vi "QuizPrimeroFinal.vi"() -> ()   [LabVIEW 2020]
panel:
  in  "?":bool
  out "El contador se encuentra":dbl
  out "LED3":bool
  out "LED2":bool
  out "LED1":bool
  out "SW/CO":bool
  out "Led Tres":bool
  out "Led Dos":bool
  out "Led Uno":bool
  in  "Pulsador Tres":bool
  in  "Pulsador Dos":bool
  in  "Pulsador Uno":bool
  out "Visualizador del tiempo del contador en ms":i32
  out "Contador del sistema":dbl
  out "Respuesta de la trama":string
  in  "Ingrese la trama completa":string
  in  "Botón ENTER":bool
  out "Respuesta de comandos":string
  out "Opción":i8
  in  "Ingrese comando":string
  # "Comandos AT"
  # "Indicadores"
  # "Botón STOP"
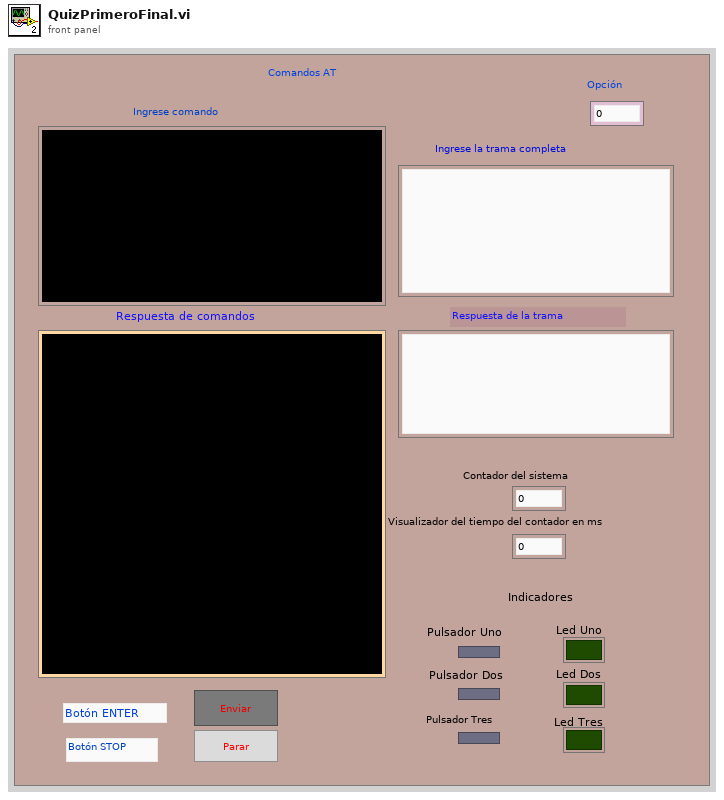
[diagram p1: front panel]
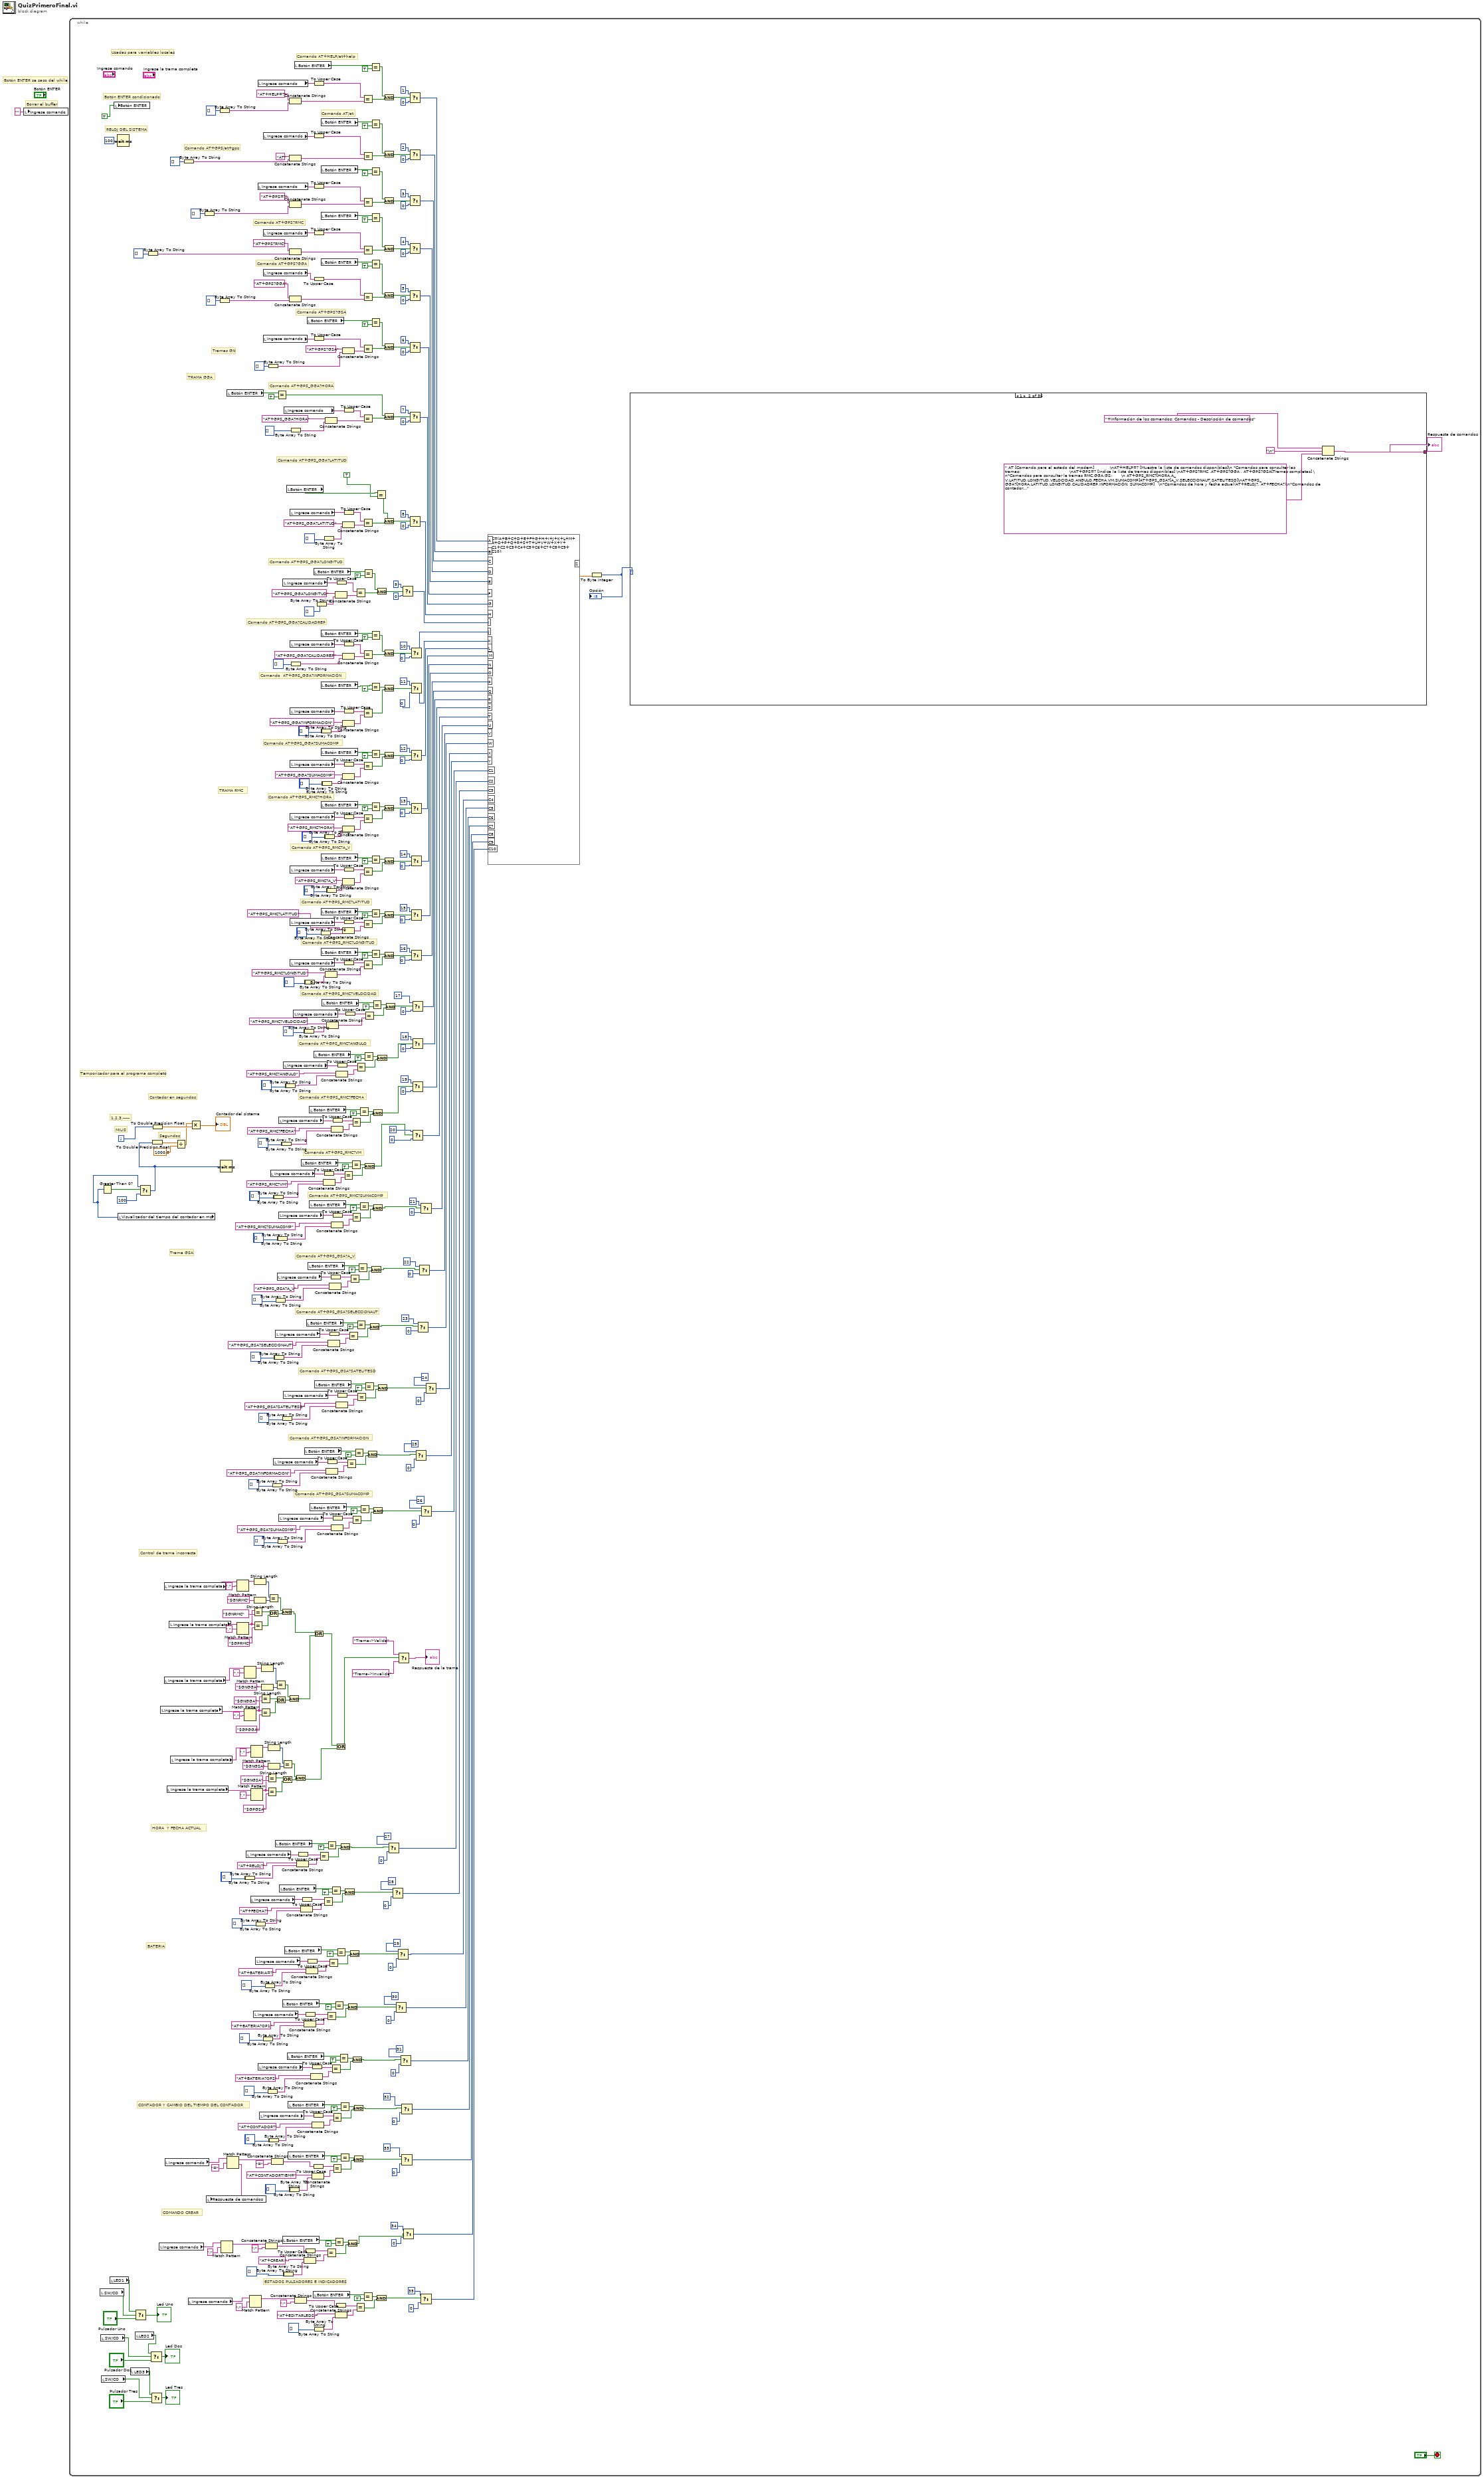
[diagram p0: block diagram]
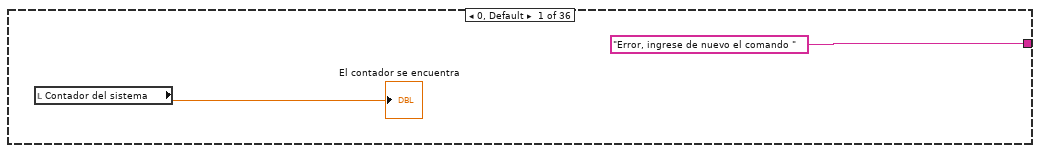
[diagram p2: hidden frame]
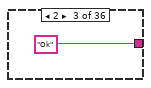
[diagram p3: hidden frame]
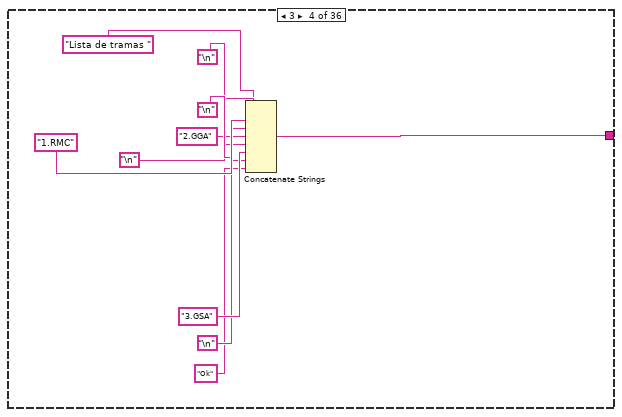
[diagram p4: hidden frame]
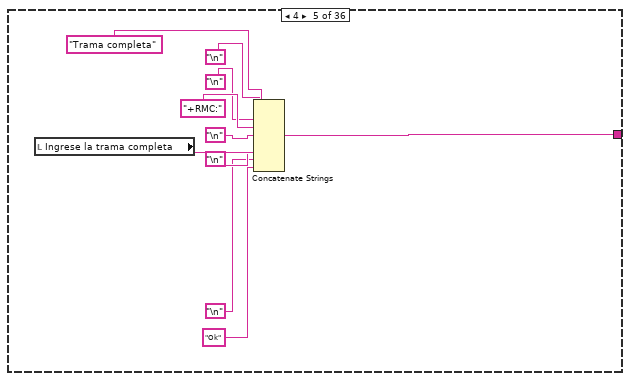
[diagram p5: hidden frame]
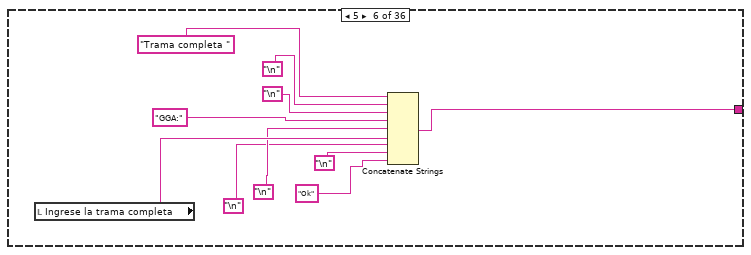
[diagram p6: hidden frame]
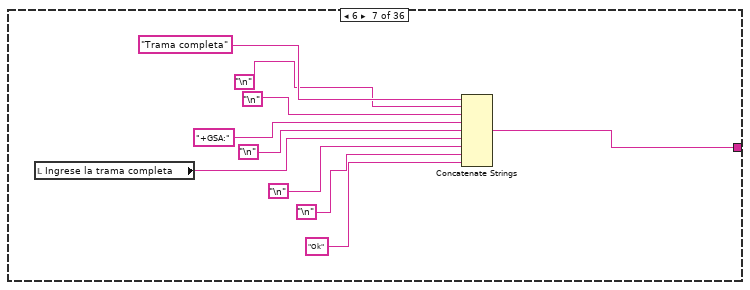
[diagram p7: hidden frame]
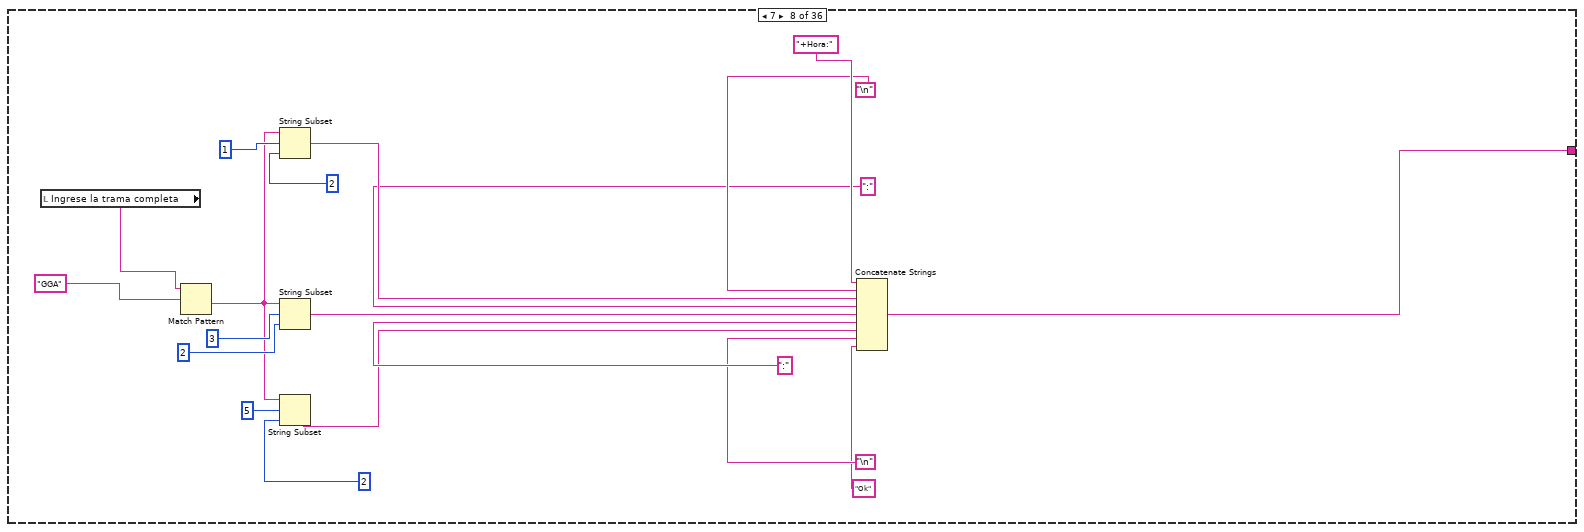
[diagram p8: hidden frame]
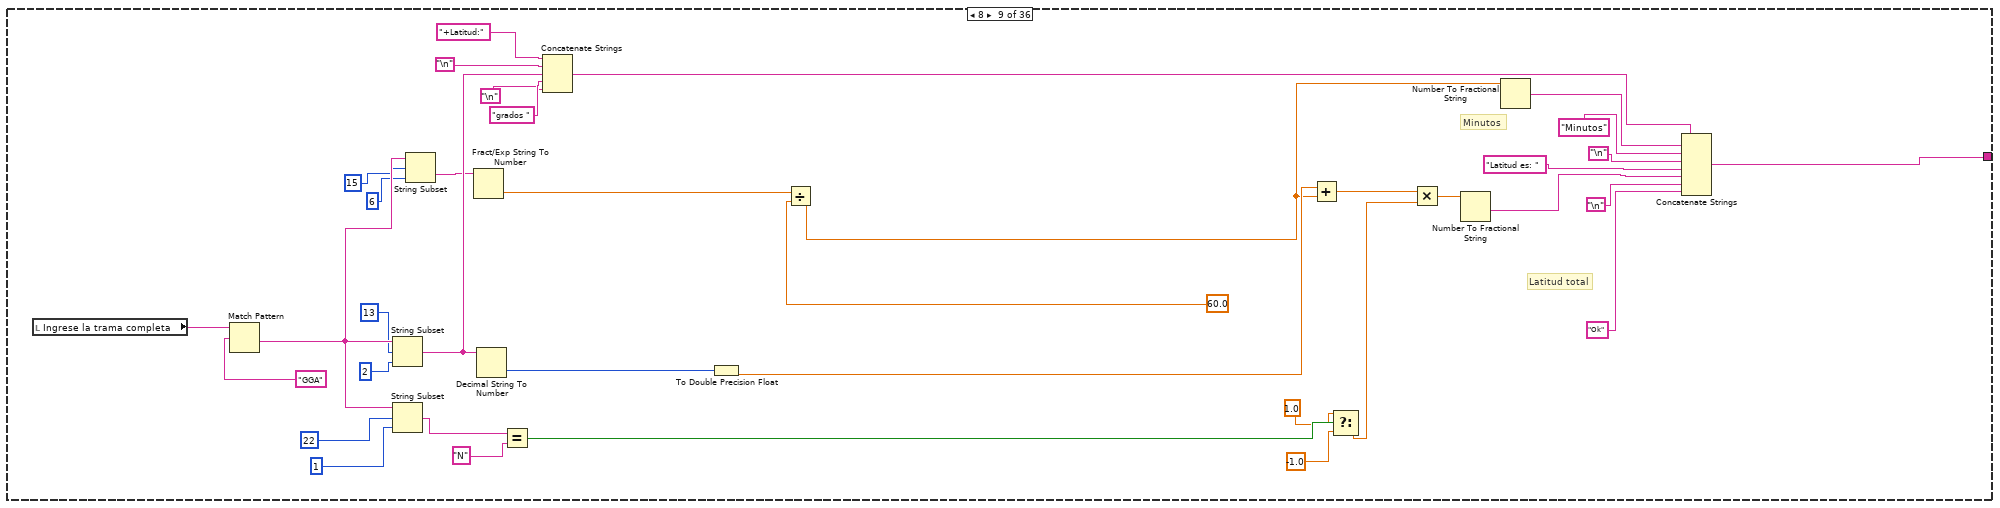
[diagram p9: hidden frame]
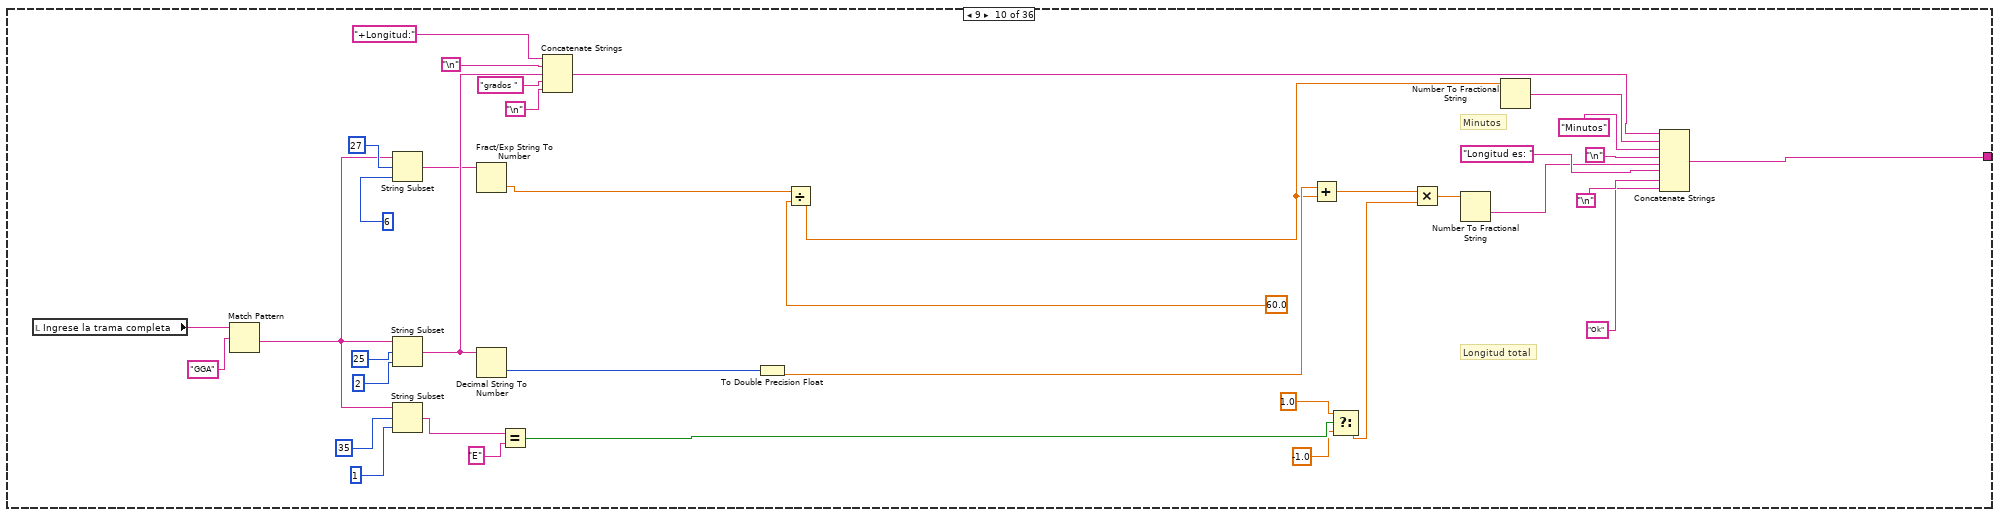
[diagram p10: hidden frame]
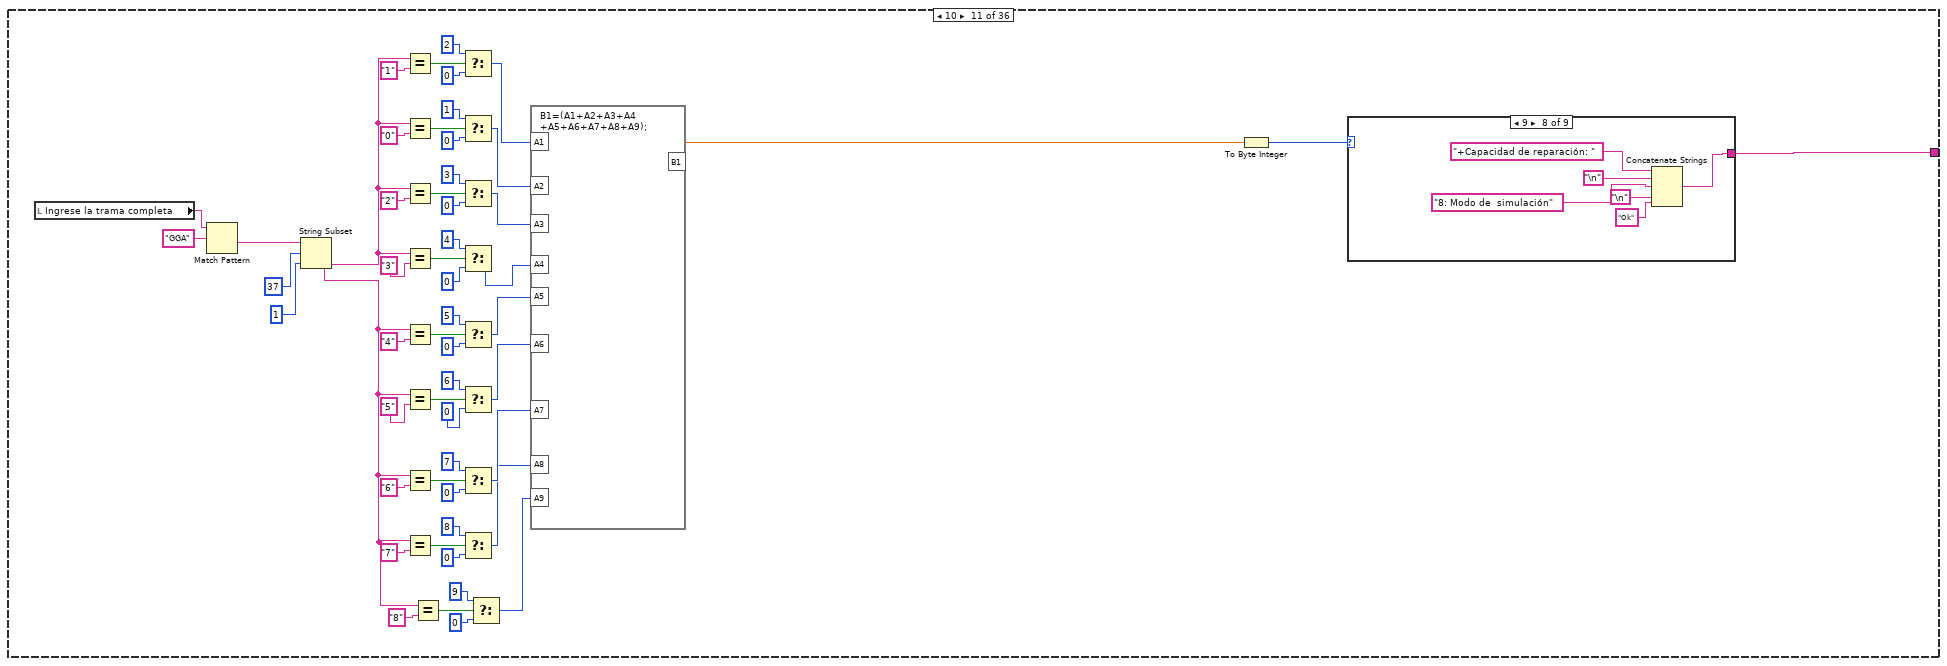
[diagram p11: hidden frame]
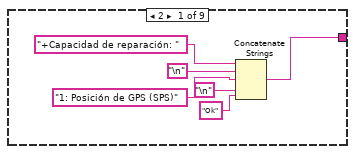
[diagram p12: hidden frame]
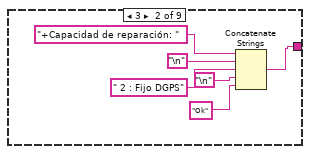
[diagram p13: hidden frame]
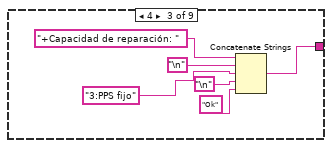
[diagram p14: hidden frame]
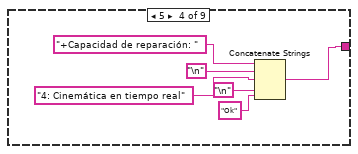
[diagram p15: hidden frame]
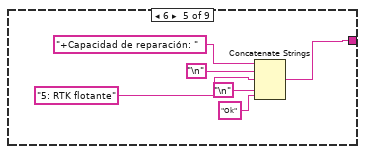
[diagram p16: hidden frame]
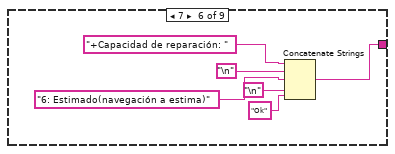
[diagram p17: hidden frame]
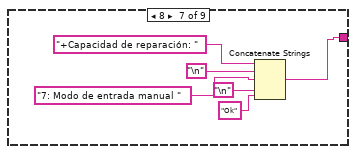
[diagram p18: hidden frame]
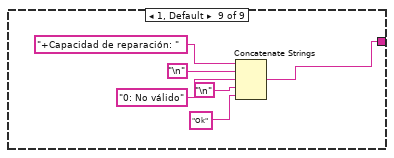
[diagram p19: hidden frame]
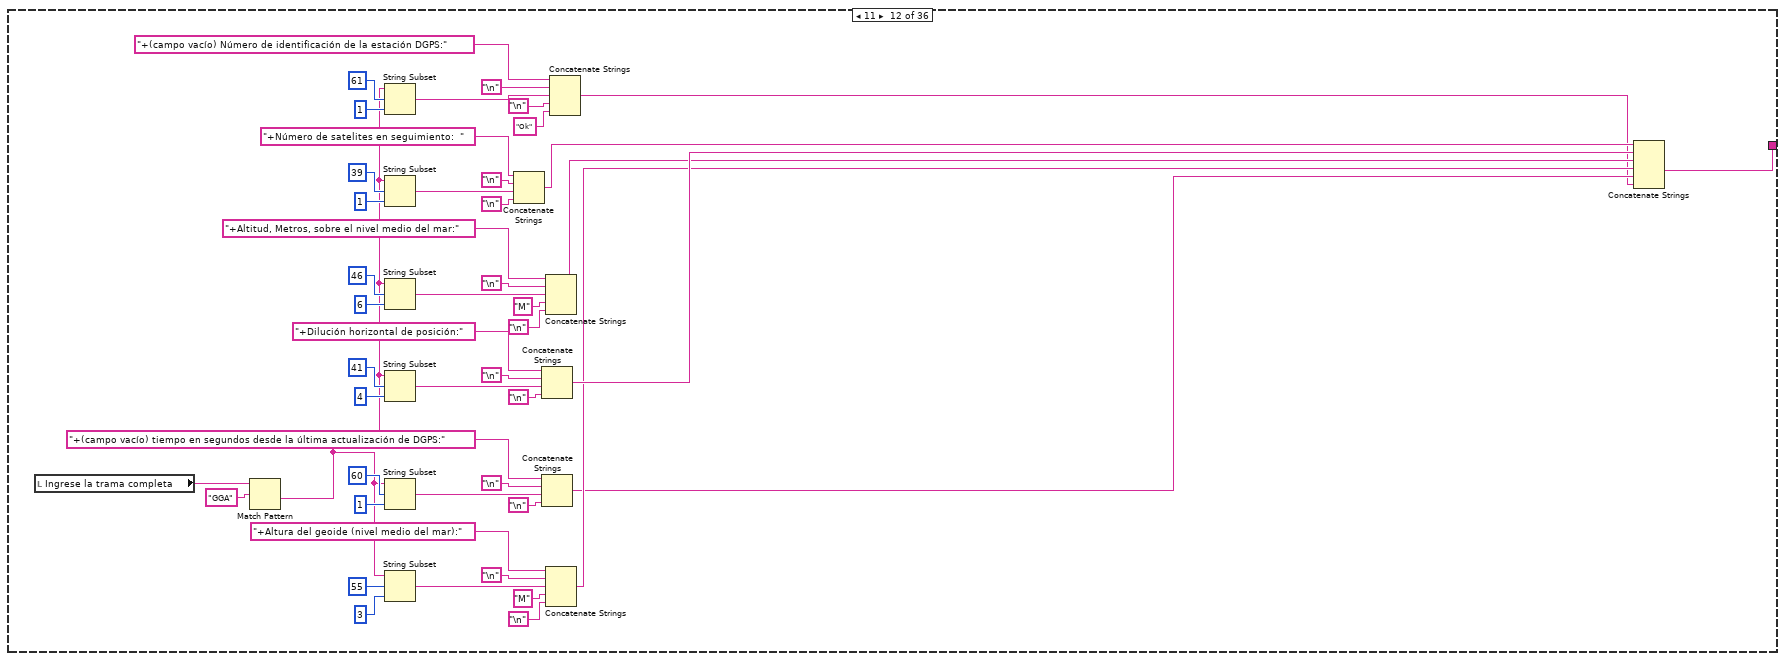
[diagram p20: hidden frame]
diagram:
  # "Botón ENTER se saco del while"
  # "Borrar el buffer"
  n1 = local write "Ingrese comando"("" ("Ingrese comando")) -> ()
  n2 = while {
    i -> [w63]
    stop <- "?" stop-if-true
    # "RELOJ DEL SISTEMA"
    # "Botón ENTER condicionado"
    # "Temporizador para el programa completo"
    # "COMANDO CREAR"
    # "ESTADOS PULSADORES E INDICADORES"
    # "Segundos"
    # "MILIS"
    # "1,2,3,-----"
    # "CONTADOR Y CAMBIO DEL TIEMPO DEL CONTADOR"
    # "BATERIA"
    # "HORA  Y FECHA ACTUAL"
    # "Tramas GN"
    # "Control de trama incorrecta"
    # "Comando AT+GPS_GSA?SUMACOMP"
    # "Comando AT+GPS_GSA?INFORMACION"
    # "Comando AT+GPS_GSA?SATELITESD"
    # "Comando AT+GPS_GSA?SELECCIONAUT"
    # "Comando AT+GPS_GSA?A_V"
    # "Trama GSA"
    # "Comando AT+GPS_RMC?SUMACOMP"
    # "Comando AT+GPS_RMC?VM"
    # "Comando AT+GPS_RMC?FECHA"
    # "Comando AT+GPS_RMC?ANGULO"
    # "Comando AT+GPS_RMC?VELOCIDAD"
    # "TRAMA RMC"
    # "Contador en segundos"
    # "Comando AT+GPS_RMC?LONGITUD"
    # "Comando AT+GPS_RMC?A_V"
    # "TRAMA GGA"
    # "Comando AT+GPS_RMC?LATITUD"
    # "Comando AT+GPS_RMC?HORA"
    # "Comando AT+GPS_GGA?SUMACOMP"
    # "Comando  AT+GPS_GGA?INFORMACIÓN"
    # "Comando AT+GPS_GGA?CALIDADREP"
    # "Comando AT+GPS_GGA?LONGITUD"
    # "Usadas para varriables locales"
    # "Comando AT+GPS_GGA?LATITUD"
    # "Comando AT+GPS_GGA?HORA"
    # "Comando AT+GPS?GSA"
    # "Comando AT+GPS?GGA"
    # "Comando AT+GPS?RMC"
    # "Comando AT+HELP/at+help"
    # "Comando AT+GPS/at+gps"
    # "Comando AT/at"
    n3 = local read "SW/CO"() -> (w30:bool)
    n4 = local read "SW/CO"() -> (w29:bool)
    n5 = local read "SW/CO"() -> (w50:bool)
    n6 = local read "LED1"() -> (w28:bool)
    n7 = local write "Botón ENTER"(TRUE ("Botón ENTER")) -> ()
    n8 = Wait (ms)(milliseconds to wait=u32 100) -> ()  [unwired: 1 out]
    n9 = local read "Visualizador del tiempo del contador en ms"() -> (w5:i32)
    n10 = Greater Than 0?(x=w5) -> (x > 0?=w6:bool)
    n11 = local read "LED3"() -> (w26:bool)
    n12 = Select(t=w28, s=w30, f="Pulsador Uno") -> (s? t:f=→"Led Uno":bool)
    n13 = local read "LED2"() -> (w27:bool)
    n14 = Select(t=w5, s=w6, f=100) -> (s? t:f=w3:i32)
    n15 = Byte Array To String(unsigned byte array=u8[] []) -> (string=w380:string)
    n16 = Select(t=w27, s=w29, f="Pulsador Dos") -> (s? t:f=→"Led Dos":bool)
    n17 = Select(t=w26, s=w50, f="Pulsador Tres") -> (s? t:f=→"Led Tres":bool)
    n18 = To Double Precision Float(number=w3) -> (double precision float=w62:dbl)
    n19 = To Double Precision Float(number=w63) -> (double precision float=w84:dbl)
    n20 = local read "Ingrese comando"() -> (w13:string)
    n21 = local read "Ingrese la trama completa"() -> (w198:string)
    n22 = local read "Ingrese la trama completa"() -> (w193:string)
    n23 = local read "Ingrese la trama completa"() -> (w197:string)
    n24 = local read "Ingrese comando"() -> (w69:string)
    n25 = local read "Ingrese la trama completa"() -> (w191:string)
    n26 = local read "Ingrese la trama completa"() -> (w217:string)
    n27 = local read "Ingrese la trama completa"() -> (w192:string)
    n28 = Divide(x=w62, y=1000.0) -> (x/y=w60:dbl)
    n29 = Byte Array To String(unsigned byte array=u8[] []) -> (string=w384:string)
    n30 = local read "Ingrese comando"() -> (w45:string)
    n31 = Multiply(x=w60, y=w84) -> (x*y=→"Contador del sistema":dbl)
    n32 = Byte Array To String(unsigned byte array=u8[] []) -> (string=w382:string)
    n33 = Byte Array To String(unsigned byte array=u8[] []) -> (string=w387:string)
    n34 = Byte Array To String(unsigned byte array=u8[] []) -> (string=w378:string)
    n35 = Wait (ms)(milliseconds to wait=w3) -> ()  [unwired: 1 out]
    n36 = Match Pattern(string=w13, regular expression=":") -> (before substring=w11:string)  [unwired: 1 in, 3 out]
    n37 = Match Pattern(string=w69, regular expression="=") -> (before substring=w67:string, after substring=w64:string)  [unwired: 1 in, 2 out]
    n38 = local write "Respuesta de comandos"(w64) -> ()
    n39 = local read "Botón ENTER"() -> (w534:bool)
    n40 = Match Pattern(string=w193, regular expression=",") -> (before substring=w224:string)  [unwired: 1 in, 3 out]
    n41 = Match Pattern(string=w217, regular expression=",") -> (before substring=w215:string)  [unwired: 1 in, 3 out]
    n42 = Byte Array To String(unsigned byte array=u8[] []) -> (string=w162:string)
    n43 = Byte Array To String(unsigned byte array=u8[] []) -> ()  [unwired: 1 out]
    n44 = Match Pattern(string=w197, regular expression=",") -> (before substring=w204:string)  [unwired: 1 in, 3 out]
    n45 = Match Pattern(string=w198, regular expression=",") -> (before substring=w212:string)  [unwired: 1 in, 3 out]
    n46 = local read "Ingrese comando"() -> (w173:string)
    n47 = Match Pattern(string=w45, regular expression=":") -> (before substring=w47:string)  [unwired: 1 in, 3 out]
    n48 = local read "Ingrese comando"() -> (w150:string)
    n49 = Match Pattern(string=w192, regular expression=",") -> (before substring=w187:string)  [unwired: 1 in, 3 out]
    n50 = Match Pattern(string=w191, regular expression=",") -> (before substring=w179:string)  [unwired: 1 in, 3 out]
    n51 = Equal?(x=w215, y="$GNRMC") -> (x = y?=w219:bool)
    n52 = Equal?(x=w215, y="$GPRMC") -> (x = y?=w218:bool)
    n53 = local read "Ingrese comando"() -> (w125:string)
    n54 = String Length(string=w224) -> (length=w223:i32)
    n55 = String Length(string="$GNRMC" ("y")) -> (length=w226:i32)
    n56 = Byte Array To String(unsigned byte array=u8[] []) -> (string=w145:string)
    n57 = Byte Array To String(unsigned byte array=u8[] []) -> ()  [unwired: 1 out]
    n58 = local read "Ingrese comando"() -> (w135:string)
    n59 = local read "Ingrese comando"() -> (w598:string)
    n60 = local read "Ingrese comando"() -> (w605:string)
    n61 = local read "Ingrese comando"() -> (w106:string)
    n62 = local read "Ingrese comando"() -> (w96:string)
    n63 = Equal?(x=w212, y="$GNGGA") -> (x = y?=w209:bool)
    n64 = Equal?(x=w212, y="$GPGGA") -> (x = y?=w210:bool)
    n65 = String Length(string=w204) -> (length=w205:i32)
    n66 = String Length(string="$GNGGA" ("y")) -> (length=w202:i32)
    n67 = Byte Array To String(unsigned byte array=u8[] []) -> (string=w129:string)
    n68 = Byte Array To String(unsigned byte array=u8[] []) -> ()  [unwired: 1 out]
    n69 = local read "Ingrese comando"() -> (w526:string)
    n70 = local read "Ingrese comando"() -> (w572:string)
    n71 = local read "Ingrese comando"() -> (w562:string)
    n72 = local read "Ingrese comando"() -> (w550:string)
    n73 = Byte Array To String(unsigned byte array=u8[] []) -> (string=w131:string)
    n74 = Byte Array To String(unsigned byte array=u8[] []) -> ()  [unwired: 1 out]
    n75 = Concatenate Strings(w11, ":" ("string")) -> (w9:string)
    n76 = Equal?(x=w179, y="$GNGSA") -> (x = y?=w182:bool)
    n77 = Equal?(x=w179, y="$GPGSA") -> (x = y?=w181:bool)
    n78 = Byte Array To String(unsigned byte array=u8[] []) -> (string=w102:string)
    n79 = Byte Array To String(unsigned byte array=u8[] []) -> ()  [unwired: 1 out]
    n80 = Byte Array To String(unsigned byte array=u8[] []) -> (string=w376:string)
    n81 = Byte Array To String(unsigned byte array=u8[] []) -> (string=w99:string)
    n82 = Equal?(x=w223, y=w226) -> (x = y?=w222:bool)
    n83 = Or(x=w219, y=w218) -> (x .or. y?=w214:bool)
    n84 = String Length(string=w187) -> (length=w186:i32)
    n85 = String Length(string="$GNGSA" ("y")) -> (length=w189:i32)
    n86 = Byte Array To String(unsigned byte array=u8[] []) -> ()  [unwired: 1 out]
    n87 = local read "Ingrese comando"() -> (w321:string)
    n88 = Byte Array To String(unsigned byte array=u8[] []) -> (string=w246:string)
    n89 = Byte Array To String(unsigned byte array=u8[] []) -> ()  [unwired: 1 out]
    n90 = Concatenate Strings(w67, "=" ("string")) -> (w65:string)
    n91 = Byte Array To String(unsigned byte array=u8[] []) -> (string=w331:string)
    n92 = Byte Array To String(unsigned byte array=u8[] []) -> ()  [unwired: 1 out]
    n93 = Byte Array To String(unsigned byte array=u8[] []) -> (string=w276:string)
    n94 = Byte Array To String(unsigned byte array=u8[] []) -> ()  [unwired: 1 out]
    n95 = local read "Ingrese comando"() -> (w257:string)
    n96 = Byte Array To String(unsigned byte array=u8[] []) -> (string=w303:string)
    n97 = Byte Array To String(unsigned byte array=u8[] []) -> ()  [unwired: 1 out]
    n98 = Equal?(x=w205, y=w202) -> (x = y?=w206:bool)
    n99 = Or(x=w209, y=w210) -> (x .or. y?=w213:bool)
    n100 = local read "Botón ENTER"() -> (w169:bool)
    n101 = local read "Ingrese comando"() -> (w287:string)
    n102 = Byte Array To String(unsigned byte array=u8[] []) -> (string=w308:string)
    n103 = Equal?(x=w534, y=TRUE) -> (x = y?=w535:bool)
    n104 = Byte Array To String(unsigned byte array=u8[] []) -> ()  [unwired: 1 out]
    n105 = Byte Array To String(unsigned byte array=u8[] []) -> (string=w242:string)
    n106 = Byte Array To String(unsigned byte array=u8[] []) -> ()  [unwired: 1 out]
    n107 = local read "Ingrese comando"() -> (w292:string)
    n108 = local read "Ingrese comando"() -> (w343:string)
    n109 = local read "Ingrese comando"() -> (w319:string)
    n110 = local read "Ingrese comando"() -> (w231:string)
    n111 = local read "Botón ENTER"() -> (w154:bool)
    n112 = Byte Array To String(unsigned byte array=u8[] []) -> (string=w332:string)
    n113 = Byte Array To String(unsigned byte array=u8[] []) -> ()  [unwired: 1 out]
    n114 = Byte Array To String(unsigned byte array=u8[] []) -> (string=w272:string)
    n115 = And(x=w222, y=w214) -> (x .and. y?=w195:bool)
    n116 = Byte Array To String(unsigned byte array=u8[] []) -> ()  [unwired: 1 out]
    n117 = Equal?(x=w186, y=w189) -> (x = y?=w185:bool)
    n118 = Or(x=w182, y=w181) -> (x .or. y?=w178:bool)
    n119 = Byte Array To String(unsigned byte array=u8[] []) -> (string=w14:string)
    n120 = local read "Botón ENTER"() -> (w121:bool)
    n121 = local read "Botón ENTER"() -> (w20:bool)
    n122 = Byte Array To String(unsigned byte array=u8[] []) -> ()  [unwired: 1 out]
    n123 = local read "Ingrese comando"() -> (w513:string)
    n124 = local read "Ingrese comando"() -> (w396:string)
    n125 = local read "Ingrese comando"() -> (w261:string)
    n126 = local read "Ingrese comando"() -> (w539:string)
    n127 = Byte Array To String(unsigned byte array=u8[] []) -> (string=w344:string)
    n128 = Byte Array To String(unsigned byte array=u8[] []) -> ()  [unwired: 1 out]
    n129 = local read "Botón ENTER"() -> (w139:bool)
    n130 = local read "Botón ENTER"() -> (w520:bool)
    n131 = local read "Botón ENTER"() -> (w110:bool)
    n132 = Byte Array To String(unsigned byte array=u8[] []) -> (string=w70:string)
    n133 = And(x=w206, y=w213) -> (x .and. y?=w194:bool)
    n134 = local read "Botón ENTER"() -> (w92:bool)
    n135 = local read "Botón ENTER"() -> (w78:bool)
    n136 = Byte Array To String(unsigned byte array=u8[] []) -> ()  [unwired: 1 out]
    n137 = Concatenate Strings "Concatenate Strings"("AT+HELP=?" ("string"), w387) -> (w597:string)
    n138 = Concatenate Strings "Concatenate Strings"("AT" ("y"), w384) -> (w607:string)
    n139 = Concatenate Strings "Concatenate Strings"("AT+GPS=?" ("string"), w382) -> (w603:string)
    n140 = Concatenate Strings "Concatenate Strings"("AT+GPS?RMC" ("string"), w380) -> (w574:string)
    n141 = Concatenate Strings "Concatenate Strings"("AT+GPS?GGA" ("string"), w378) -> (w559:string)
    n142 = Byte Array To String(unsigned byte array=u8[] []) -> (string=w374:string)
    n143 = Byte Array To String(unsigned byte array=u8[] []) -> (string=w368:string)
    n144 = local read "Ingrese comando"() -> (w524:string)
    n145 = local read "Ingrese comando"() -> (w491:string)
    n146 = local read "Ingrese comando"() -> (w489:string)
    n147 = local read "Ingrese comando"() -> (w467:string)
    n148 = local read "Ingrese comando"() -> (w465:string)
    n149 = local read "Ingrese comando"() -> (w443:string)
    n150 = local read "Ingrese comando"() -> (w441:string)
    n151 = local read "Ingrese comando"() -> (w419:string)
    n152 = local read "Ingrese comando"() -> (w417:string)
    n153 = local read "Botón ENTER"() -> (w581:bool)
    n154 = Concatenate Strings(w47, ":" ("string")) -> (w49:string)
    n155 = And(x=w185, y=w178) -> (x .and. y?=w177:bool)
    n156 = Concatenate Strings("AT+RELOJ?" ("string"), w162) -> (w170:string)
    n157 = To Upper Case(1:w173) -> (0:w172:string)
    n158 = Concatenate Strings("AT+FECHA?" ("string"), w145) -> (w153:string)
    n159 = local read "Botón ENTER"() -> (w325:bool)
    n160 = To Upper Case(1:w150) -> (0:w151:string)
    n161 = Byte Array To String(unsigned byte array=u8[] []) -> (string=w347:string)
    n162 = Byte Array To String(unsigned byte array=u8[] []) -> ()  [unwired: 1 out]
    n163 = Byte Array To String(unsigned byte array=u8[] []) -> (string=w348:string)
    n164 = Byte Array To String(unsigned byte array=u8[] []) -> ()  [unwired: 1 out]
    n165 = Concatenate Strings("AT+BATERIA?OP1" ("string"), w129) -> (w122:string)
    n166 = Concatenate Strings("AT+CREAR:" ("string"), w14) -> (w19:string)
    n167 = local read "Botón ENTER"() -> (w253:bool)
    n168 = To Upper Case(1:w125) -> (0:w124:string)
    n169 = To Upper Case(1:w9) -> (0:w17:string)
    n170 = Concatenate Strings("AT+BATERIA=?" ("string"), w131) -> (w138:string)
    n171 = local read "Botón ENTER"() -> (w283:bool)
    n172 = To Upper Case(1:w135) -> (0:w136:string)
    n173 = local read "Botón ENTER"() -> (w547:bool)
    n174 = local read "Botón ENTER"() -> (w296:bool)
    n175 = local read "Botón ENTER"() -> (w339:bool)
    n176 = local read "Botón ENTER"() -> (w315:bool)
    n177 = local read "Botón ENTER"() -> (w235:bool)
    n178 = Concatenate Strings("AT+BATERIA?OP2" ("string"), w102) -> (w109:string)
    n179 = To Upper Case(1:w106) -> (0:w107:string)
    n180 = Concatenate Strings("AT+CONTADOR?" ("string"), w99) -> (w93:string)
    n181 = Concatenate Strings("AT+CONTADORTIEM=" ("string"), w70) -> (w77:string)
    n182 = To Upper Case(1:w96) -> (0:w95:string)
    n183 = To Upper Case(1:w65) -> (0:w75:string)
    n184 = To Upper Case(1:w598) -> (0:w596:string)
    n185 = To Upper Case(1:w526) -> (0:w608:string)
    n186 = To Upper Case(1:w605) -> (0:w606:string)
    n187 = To Upper Case(1:w572) -> (0:w571:string)
    n188 = To Upper Case(1:w562) -> (0:w561:string)
    n189 = To Upper Case(1:w550) -> (0:w551:string)
    n190 = Byte Array To String(unsigned byte array=u8[] []) -> (string=w44:string)
    n191 = Or(x=w195, y=w194) -> (x .or. y?=w176:bool)
    n192 = local read "Botón ENTER"() -> (w38:bool)
    n193 = Byte Array To String(unsigned byte array=u8[] []) -> ()  [unwired: 1 out]
    n194 = local read "Botón ENTER"() -> (w509:bool)
    n195 = local read "Botón ENTER"() -> (w400:bool)
    n196 = local read "Botón ENTER"() -> (w265:bool)
    n197 = Byte Array To String(unsigned byte array=u8[] []) -> (string=w370:string)
    n198 = Equal?(x=w172, y=w170) -> (x = y?=w166:bool)
    n199 = Byte Array To String(unsigned byte array=u8[] []) -> (string=w349:string)
    n200 = Byte Array To String(unsigned byte array=u8[] []) -> (string=w359:string)
    n201 = Byte Array To String(unsigned byte array=u8[] []) -> ()  [unwired: 1 out]
    n202 = Byte Array To String(unsigned byte array=u8[] []) -> ()  [unwired: 1 out]
    n203 = Byte Array To String(unsigned byte array=u8[] []) -> (string=w358:string)
    n204 = local read "Botón ENTER"() -> (w525:bool)
    n205 = local read "Botón ENTER"() -> (w586:bool)
    n206 = local read "Botón ENTER"() -> (w570:bool)
    n207 = local read "Botón ENTER"() -> (w558:bool)
    n208 = local read "Botón ENTER"() -> (w495:bool)
    n209 = local read "Botón ENTER"() -> (w485:bool)
    n210 = local read "Botón ENTER"() -> (w471:bool)
    n211 = Byte Array To String(unsigned byte array=u8[] []) -> ()  [unwired: 1 out]
    n212 = local read "Botón ENTER"() -> (w461:bool)
    n213 = local read "Botón ENTER"() -> (w447:bool)
    n214 = local read "Botón ENTER"() -> (w437:bool)
    n215 = local read "Botón ENTER"() -> (w423:bool)
    n216 = local read "Botón ENTER"() -> (w413:bool)
    n217 = Equal?(x=w151, y=w153) -> (x = y?=w157:bool)
    n218 = Byte Array To String(unsigned byte array=u8[] []) -> (string=w372:string)
    n219 = Concatenate Strings("AT+GPS_RMC?VM" ("string"), w331) -> (w324:string)
    n220 = Byte Array To String(unsigned byte array=u8[] []) -> (string=w357:string)
    n221 = To Upper Case(1:w321) -> (0:w322:string)
    n222 = Byte Array To String(unsigned byte array=u8[] []) -> ()  [unwired: 1 out]
    n223 = Concatenate Strings("AT+GPS_GGA?HORA" ("string"), w374) -> (w537:string)
    n224 = Byte Array To String(unsigned byte array=u8[] []) -> (string=w356:string)
    n225 = Concatenate Strings("AT+GPS_RMC?LONGITUD" ("string"), w348) -> (w422:string)
    n226 = Byte Array To String(unsigned byte array=u8[] []) -> ()  [unwired: 1 out]
    n227 = Equal?(x=w124, y=w122) -> (x = y?=w118:bool)
    n228 = Equal?(x=w17, y=w19) -> (x = y?=w23:bool)
    n229 = Concatenate Strings("AT+GPS_GSA?INFORMACION" ("string"), w246) -> (w254:string)
    n230 = Equal?(x=w169, y=TRUE) -> (x = y?=w167:bool)
    n231 = Concatenate Strings("AT+GPS_RMC?VELOCIDAD" ("string"), w347) -> (w414:string)
    n232 = To Upper Case(1:w257) -> (0:w256:string)
    n233 = Equal?(x=w136, y=w138) -> (x = y?=w142:bool)
    n234 = Concatenate Strings("AT+GPS_GSA?SELECCIONAUT" ("string"), w276) -> (w284:string)
    n235 = To Upper Case(1:w287) -> (0:w286:string)
    n236 = Concatenate Strings("AT+GPS_GSA?A_V" ("string"), w303) -> (w295:string)
    n237 = To Upper Case(1:w292) -> (0:w293:string)
    n238 = Equal?(x=w154, y=TRUE) -> (x = y?=w156:bool)
    n239 = Equal?(x=w107, y=w109) -> (x = y?=w113:bool)
    n240 = Concatenate Strings("AT+GPS_RMC?FECHA" ("string"), w332) -> (w340:string)
    n241 = Concatenate Strings("AT+GPS_RMC?SUMACOMP" ("string"), w308) -> (w316:string)
    n242 = To Upper Case(1:w343) -> (0:w342:string)
    n243 = To Upper Case(1:w319) -> (0:w318:string)
    n244 = Concatenate Strings("AT+GPS_GSA?SUMACOMP" ("string"), w242) -> (w234:string)
    n245 = Equal?(x=w95, y=w93) -> (x = y?=w89:bool)
    n246 = Equal?(x=w75, y=w77) -> (x = y?=w81:bool)
    n247 = To Upper Case(1:w231) -> (0:w232:string)
    n248 = Equal?(x=w121, y=TRUE) -> (x = y?=w119:bool)
    n249 = Equal?(x=w20, y=TRUE) -> (x = y?=w22:bool)
    n250 = Concatenate Strings("AT+EDITARLEDS:" ("string"), w44) -> (w39:string)
    n251 = Concatenate Strings("AT+GPS_GGA?LONGITUD" ("string"), w370) -> (w510:string)
    n252 = Or(x=w176, y=w177) -> (x .or. y?=w175:bool)
    n253 = Equal?(x=w139, y=TRUE) -> (x = y?=w141:bool)
    n254 = To Upper Case(1:w49) -> (0:w41:string)
    n255 = To Upper Case(1:w513) -> (0:w512:string)
    n256 = Concatenate Strings("AT+GPS_RMC?ANGULO" ("string"), w344) -> (w399:string)
    n257 = To Upper Case(1:w396) -> (0:w397:string)
    n258 = Concatenate Strings("AT+GPS_GSA?SATELITESD" ("string"), w272) -> (w264:string)
    n259 = To Upper Case(1:w261) -> (0:w262:string)
    n260 = Equal?(x=w110, y=TRUE) -> (x = y?=w112:bool)
    n261 = Equal?(x=w92, y=TRUE) -> (x = y?=w90:bool)
    n262 = Equal?(x=w78, y=TRUE) -> (x = y?=w80:bool)
    n263 = And(x=w167, y=w166) -> (x .and. y?=w165:bool)
    n264 = Concatenate Strings("AT+GPS?GSA" ("string"), w376) -> (w549:string)
    n265 = Concatenate Strings("AT+GPS_GGA?LATITUD" ("string"), w372) -> (w522:string)
    n266 = Concatenate Strings("AT+GPS_GGA?CALIDADREP" ("string"), w368) -> (w494:string)
    n267 = Concatenate Strings("AT+GPS_GGA?INFORMACION" ("string"), w359) -> (w486:string)
    n268 = Concatenate Strings("AT+GPS_GGA?SUMACOMP" ("string"), w358) -> (w470:string)
    n269 = Concatenate Strings("AT+GPS_RMC?HORA" ("string"), w357) -> (w462:string)
    n270 = Concatenate Strings("AT+GPS_RMC?A_V" ("string"), w356) -> (w446:string)
    n271 = Concatenate Strings("AT+GPS_RMC?LATITUD" ("string"), w349) -> (w438:string)
    n272 = Equal?(x=w322, y=w324) -> (x = y?=w328:bool)
    n273 = To Upper Case(1:w539) -> (0:w538:string)
    n274 = To Upper Case(1:w524) -> (0:w523:string)
    n275 = To Upper Case(1:w491) -> (0:w492:string)
    n276 = To Upper Case(1:w489) -> (0:w488:string)
    n277 = To Upper Case(1:w467) -> (0:w468:string)
    n278 = To Upper Case(1:w465) -> (0:w464:string)
    n279 = To Upper Case(1:w443) -> (0:w444:string)
    n280 = To Upper Case(1:w441) -> (0:w440:string)
    n281 = To Upper Case(1:w419) -> (0:w420:string)
    n282 = And(x=w156, y=w157) -> (x .and. y?=w158:bool)
    n283 = To Upper Case(1:w417) -> (0:w416:string)
    n284 = Equal?(x=w256, y=w254) -> (x = y?=w250:bool)
    n285 = And(x=w119, y=w118) -> (x .and. y?=w117:bool)
    n286 = And(x=w22, y=w23) -> (x .and. y?=w8:bool)
    n287 = Equal?(x=w286, y=w284) -> (x = y?=w280:bool)
    n288 = And(x=w141, y=w142) -> (x .and. y?=w143:bool)
    n289 = Equal?(x=w293, y=w295) -> (x = y?=w299:bool)
    n290 = Equal?(x=w325, y=TRUE) -> (x = y?=w327:bool)
    n291 = Equal?(x=w342, y=w340) -> (x = y?=w336:bool)
    n292 = Equal?(x=w318, y=w316) -> (x = y?=w312:bool)
    n293 = Equal?(x=w232, y=w234) -> (x = y?=w238:bool)
    n294 = And(x=w112, y=w113) -> (x .and. y?=w114:bool)
    n295 = And(x=w90, y=w89) -> (x .and. y?=w88:bool)
    n296 = And(x=w80, y=w81) -> (x .and. y?=w82:bool)
    n297 = Equal?(x=w253, y=TRUE) -> (x = y?=w251:bool)
    n298 = Equal?(x=w41, y=w39) -> (x = y?=w35:bool)
    n299 = Equal?(x=w512, y=w510) -> (x = y?=w506:bool)
    n300 = Equal?(x=w397, y=w399) -> (x = y?=w403:bool)
    n301 = Equal?(x=w283, y=TRUE) -> (x = y?=w281:bool)
    n302 = Equal?(x=w262, y=w264) -> (x = y?=w268:bool)
    n303 = Equal?(x=w296, y=TRUE) -> (x = y?=w298:bool)
    n304 = Equal?(x=w339, y=TRUE) -> (x = y?=w337:bool)
    n305 = Equal?(x=w315, y=TRUE) -> (x = y?=w313:bool)
    n306 = Equal?(x=w235, y=TRUE) -> (x = y?=w237:bool)
    n307 = Equal?(x=w596, y=w597) -> (x = y?=w578:bool)
    n308 = Equal?(x=w608, y=w607) -> (x = y?=w588:bool)
    n309 = Equal?(x=w606, y=w603) -> (x = y?=w583:bool)
    n310 = Equal?(x=w571, y=w574) -> (x = y?=w568:bool)
    n311 = Equal?(x=w561, y=w559) -> (x = y?=w555:bool)
    n312 = Equal?(x=w551, y=w549) -> (x = y?=w544:bool)
    n313 = Equal?(x=w538, y=w537) -> (x = y?=w528:bool)
    n314 = Equal?(x=w523, y=w522) -> (x = y?=w518:bool)
    n315 = Equal?(x=w492, y=w494) -> (x = y?=w498:bool)
    n316 = Equal?(x=w488, y=w486) -> (x = y?=w482:bool)
    n317 = Equal?(x=w468, y=w470) -> (x = y?=w474:bool)
    n318 = Equal?(x=w464, y=w462) -> (x = y?=w458:bool)
    n319 = Equal?(x=w444, y=w446) -> (x = y?=w450:bool)
    n320 = Equal?(x=w440, y=w438) -> (x = y?=w434:bool)
    n321 = Equal?(x=w420, y=w422) -> (x = y?=w426:bool)
    n322 = Equal?(x=w38, y=TRUE) -> (x = y?=w36:bool)
    n323 = Equal?(x=w509, y=TRUE) -> (x = y?=w507:bool)
    n324 = Equal?(x=w400, y=TRUE) -> (x = y?=w402:bool)
    n325 = Equal?(x=w416, y=w414) -> (x = y?=w410:bool)
    n326 = Equal?(x=w265, y=TRUE) -> (x = y?=w267:bool)
    n327 = And(x=w327, y=w328) -> (x .and. y?=w320:bool)
    n328 = And(x=w251, y=w250) -> (x .and. y?=w249:bool)
    n329 = And(x=w281, y=w280) -> (x .and. y?=w279:bool)
    n330 = Equal?(x=w581, y=TRUE) -> (x = y?=w579:bool)
    n331 = Equal?(x=w525, y=TRUE) -> (x = y?=w587:bool)
    n332 = Equal?(x=w586, y=TRUE) -> (x = y?=w584:bool)
    n333 = Equal?(x=w570, y=TRUE) -> (x = y?=w567:bool)
    n334 = Equal?(x=w558, y=TRUE) -> (x = y?=w556:bool)
    n335 = Equal?(x=w547, y=TRUE) -> (x = y?=w545:bool)
    n336 = Equal?(x=w495, y=TRUE) -> (x = y?=w497:bool)
    n337 = Equal?(x=w485, y=TRUE) -> (x = y?=w483:bool)
    n338 = Equal?(x=w471, y=TRUE) -> (x = y?=w473:bool)
    n339 = Equal?(x=w461, y=TRUE) -> (x = y?=w459:bool)
    n340 = Equal?(x=w447, y=TRUE) -> (x = y?=w449:bool)
    n341 = Equal?(x=w437, y=TRUE) -> (x = y?=w435:bool)
    n342 = Equal?(x=w423, y=TRUE) -> (x = y?=w425:bool)
    n343 = And(x=w298, y=w299) -> (x .and. y?=w300:bool)
    n344 = Equal?(x=w413, y=TRUE) -> (x = y?=w411:bool)
    n345 = And(x=w337, y=w336) -> (x .and. y?=w335:bool)
    n346 = And(x=w313, y=w312) -> (x .and. y?=w311:bool)
    n347 = And(x=w237, y=w238) -> (x .and. y?=w239:bool)
    n348 = Equal?(x=w520, y=TRUE) -> (x = y?=w519:bool)
    n349 = And(x=w36, y=w35) -> (x .and. y?=w32:bool)
    n350 = And(x=w507, y=w506) -> (x .and. y?=w505:bool)
    n351 = And(x=w402, y=w403) -> (x .and. y?=w404:bool)
    n352 = And(x=w267, y=w268) -> (x .and. y?=w269:bool)
    n353 = And(x=w579, y=w578) -> (x .and. y?=w577:bool)
    n354 = And(x=w587, y=w588) -> (x .and. y?=w589:bool)
    n355 = And(x=w584, y=w583) -> (x .and. y?=w582:bool)
    n356 = And(x=w567, y=w568) -> (x .and. y?=w566:bool)
    n357 = And(x=w556, y=w555) -> (x .and. y?=w554:bool)
    n358 = And(x=w545, y=w544) -> (x .and. y?=w543:bool)
    n359 = And(x=w535, y=w528) -> (x .and. y?=w532:bool)
    n360 = And(x=w519, y=w518) -> (x .and. y?=w517:bool)
    n361 = And(x=w497, y=w498) -> (x .and. y?=w499:bool)
    n362 = And(x=w483, y=w482) -> (x .and. y?=w481:bool)
    n363 = And(x=w473, y=w474) -> (x .and. y?=w475:bool)
    n364 = And(x=w459, y=w458) -> (x .and. y?=w457:bool)
    n365 = And(x=w449, y=w450) -> (x .and. y?=w451:bool)
    n366 = And(x=w435, y=w434) -> (x .and. y?=w433:bool)
    n367 = And(x=w425, y=w426) -> (x .and. y?=w427:bool)
    n368 = And(x=w411, y=w410) -> (x .and. y?=w409:bool)
    n369 = Select(t=27, s=w165, f=0) -> (s? t:f=w160:i32)
    n370 = Select(t=28, s=w158, f=0) -> (s? t:f=w148:i32)
    n371 = Select(t=30, s=w117, f=0) -> (s? t:f=w101:i32)
    n372 = Select(t=29, s=w143, f=0) -> (s? t:f=w130:i32)
    n373 = Select(t="Trama->Valida", s=w175, f="Trama->Invalida") -> (s? t:f=→"Respuesta de la trama":string)
    n374 = Select(t=31, s=w114, f=0) -> (s? t:f=w100:i32)
    n375 = Select(t=32, s=w88, f=0) -> (s? t:f=w85:i32)
    n376 = Select(t=33, s=w82, f=0) -> (s? t:f=w71:i32)
    n377 = Select(t=9, s=w505, f=0) -> (s? t:f=w502:i32)
    n378 = Select(t=34, s=w8, f=0) -> (s? t:f=w57:i32)
    n379 = Select(t=1, s=w577, f=0) -> (s? t:f=w575:i32)
    n380 = Select(t=i8 2, s=w589, f=i8 0) -> (s? t:f=w576:i8)
    n381 = Select(t=i8 3, s=w582, f=i8 0) -> (s? t:f=w600:i8)
    n382 = Select(t=4, s=w566, f=0) -> (s? t:f=w563:i32)
    n383 = Select(t=5, s=w554, f=0) -> (s? t:f=w552:i32)
    n384 = Select(t=6, s=w543, f=0) -> (s? t:f=w542:i32)
    n385 = Select(t=7, s=w532, f=0) -> (s? t:f=w529:i32)
    n386 = Select(t=8, s=w517, f=0) -> (s? t:f=w516:i32)
    n387 = Select(t=10, s=w499, f=0) -> (s? t:f=w490:i32)
    n388 = Select(t=11, s=w481, f=0) -> (s? t:f=w478:i32)
    n389 = Select(t=12, s=w475, f=0) -> (s? t:f=w466:i32)
    n390 = Select(t=13, s=w457, f=0) -> (s? t:f=w454:i32)
    n391 = Select(t=14, s=w451, f=0) -> (s? t:f=w442:i32)
    n392 = Select(t=15, s=w433, f=0) -> (s? t:f=w430:i32)
    n393 = Select(t=16, s=w427, f=0) -> (s? t:f=w418:i32)
    n394 = Select(t=17, s=w409, f=0) -> (s? t:f=w395:i32)
    n395 = Select(t=18, s=w404, f=0) -> (s? t:f=w394:i32)
    n396 = Select(t=19, s=w335, f=0) -> (s? t:f=w391:i32)
    n397 = Select(t=20, s=w320, f=0) -> (s? t:f=w389:i32)
    n398 = Select(t=25, s=w249, f=0) -> (s? t:f=w244:i32)
    n399 = Select(t=23, s=w279, f=0) -> (s? t:f=w274:i32)
    n400 = Select(t=22, s=w300, f=0) -> (s? t:f=w289:i32)
    n401 = Select(t=21, s=w311, f=0) -> (s? t:f=w305:i32)
    n402 = Select(t=35, s=w32, f=0) -> (s? t:f=w31:i32)
    n403 = Select(t=26, s=w239, f=0) -> (s? t:f=w229:i32)
    n404 = Select(t=24, s=w269, f=0) -> (s? t:f=w259:i32)
    n405 = formula code="Z=(A+B+C+D+E+F+G+H+I+J+K+L+M+\nN+O+P+Q+R+S+T+U+V+W+X+Y+\nC1+C2+C3+C4+C5+C6+C7+C8+C9+\nC10);"("B"=w576, "C"=w600, "A"=w575, "D"=w563, "E"=w552, "F"=w542, "G"=w529, "H"=w516, "I"=w502, "J"=w490, "K"=w478, "L"=w466, "M"=w454, "N"=w442, "O"=w430, "P"=w418, "Q"=w395, "R"=w394, "S"=w391, "T"=w389, "U"=w305, "V"=w289, "W"=w274, "X"=w259, "Y"=w244, "C1"=w229, "C2"=w160, "C3"=w148, "C4"=w130, "C5"=w101, "C6"=w100, "C7"=w85, "C8"=w71, "C9"=w57, "C10"=w31) -> ("Z"=w599:dbl)
    n406 = To Byte Integer(number=w599) -> (8bit integer=w592:i8)
    "Opción" <- w592
    n407 = case shown="1" w592 {
      tunnel: ["Error, ingrese de nuevo el comando " w616 "Ok" w618 w637 w647 w657 w668 w677 w735 w792 w894 w909 w919 w940 w955 w997 w1028 w1039 w1052 w1071 w1080 w1093 w1107 w1157 w1177 w1202 w1211 w1218 w1225 w1231 w1235 w1243 w1254 w1264 w1268] -> w228
      frame 0, Default {
        n408 = local read "Contador del sistema"() -> (→"El contador se encuentra":dbl)
      }
      frame 1 {
        n409 = Concatenate Strings "Concatenate Strings"("+Información de los comandos: Comandos - Descripción de comandos" ("string"), "\n", " AT [Comando para el estado del modem]            \nAT+HELP=? [Muestra la lista de comandos disponibles]\n *Comandos para consultar las tramas:                                     \nAT+GPS=? [Indica la lista de tramas disponibles] \nAT+GPS?RMC ,AT+GPS?GGA , AT+GPS?GSA[Tramas completas] \n*Comandos para consultar la tramas RMC,GGA,GS:       \n AT+GPS_RMC?[HORA,A_V,LATITUD,LONGITUD,VELOCIDAD,ANGULO,FECHA,VM,SUMACOMP]AT+GPS_GSA?[A_V,SELECCIONAUT,SATELITESD]\nAT+GPS_GGA?[HORA,LATITUD,LONGITUD,CALIDADREP,INFORMACIÓN, SUMACOMP]   \n*Comandos de hora y fecha actual(AT+RELOJ?, AT+FECHA?)\n*Comandos de contador y cambio de tiempo del contador(AT+CONTADOR?, AT+CONTADORTIEM=)\n*Comando bateria estática[AT+BATERIA?,AT+BATERIA?OP1,AT+BATERIA?OP2]\n*Comando para crear comando y manipulacion de leds[AT+CREAR:, AT+EDITARLEDS: SW, AT+EDITARLEDS:CO->LED1:ON,LED2:ON,LED3:ON]\n\n" ("string")) -> (w616:string)
      }
      frame 2 {
      }
      frame 3 {
        n410 = Concatenate Strings "Concatenate Strings"("Lista de tramas " ("string"), "\n", "1.RMC" ("string"), "\n", "2.GGA" ("string"), "\n", "3.GSA" ("string"), "\n", "Ok" ("string")) -> (w618:string)
      }
      frame 4 {
        n411 = local read "Ingrese la trama completa"() -> (w635:string)
        n412 = Concatenate Strings "Concatenate Strings"("Trama completa" ("string"), "\n", "\n", "+RMC:" ("string"), "\n", w635, "\n", "\n", "Ok" ("string")) -> (w637:string)
      }
      frame 5 {
        n413 = local read "Ingrese la trama completa"() -> (w646:string)
        n414 = Concatenate Strings "Concatenate Strings"("Trama completa " ("string"), "\n", "\n", "GGA:" ("string"), "\n", w646, "\n", "\n", "Ok" ("string")) -> (w647:string)
      }
      frame 6 {
        n415 = local read "Ingrese la trama completa"() -> (w651:string)
        n416 = Concatenate Strings "Concatenate Strings"("Trama completa" ("string"), "\n", "\n", "+GSA:" ("string"), "\n", w651, "\n", "\n", "Ok" ("string")) -> (w657:string)
      }
      frame 7 {
        n417 = local read "Ingrese la trama completa"() -> (w660:string)
        n418 = Match Pattern(string=w660, regular expression="GGA") -> (after substring=w671:string)  [unwired: 1 in, 3 out]
        n419 = String Subset(string=w671, offset (0)=1, length (rest)=2 ("length (rest)")) -> (substring=w665:string)
        n420 = String Subset(string=w671, offset (0)=3, length (rest)=2 ("length (rest)")) -> (substring=w663:string)
        n421 = String Subset(string=w671, offset (0)=5, length (rest)=2 ("length (rest)")) -> (substring=w661:string)
        n422 = Concatenate Strings "Concatenate Strings"("+Hora:" ("string"), "\n", w665, ":" ("string"), w663, ":" ("string"), w661, "\n", "Ok" ("string")) -> (w668:string)
      }
      frame 8 {
        # "Latitud total"
        # "Minutos"
        n423 = local read "Ingrese la trama completa"() -> (w713:string)
        n424 = Match Pattern(string=w713, regular expression="GGA") -> (after substring=w706:string)  [unwired: 1 in, 3 out]
        n425 = String Subset(string=w706, offset (0)=13, length (rest)=2 ("length (rest)")) -> (substring=w712:string)
        n426 = String Subset(string=w706, offset (0)=22, length (rest)=1 ("length (rest)")) -> (substring=w705:string)
        n427 = String Subset(string=w706, offset (0)=15, length (rest)=6 ("length (rest)")) -> (substring=w710:string)
        n428 = Fract/Exp String To Number(string=w710) -> (number=w709:dbl)  [unwired: 3 in, 1 out]
        n429 = Decimal String To Number(string=w712) -> (number=w711:i32)  [unwired: 2 in, 1 out]
        n430 = Equal?(x=w705, y="N") -> (x = y?=w704:bool)
        n431 = Concatenate Strings "Concatenate Strings"("+Latitud:" ("string"), "\n", w712, "grados " ("string"), "\n") -> (w707:string)
        n432 = To Double Precision Float(number=w711) -> (double precision float=w708:dbl)
        n433 = Divide(x=w709, y=60.0) -> (x/y=w702:dbl)
        n434 = Add(x=w708, y=w702) -> (x+y=w701:dbl)
        n435 = Select(t=1.0, s=w704, f=-1.0) -> (s? t:f=w703:dbl)
        n436 = Multiply(x=w701, y=w703) -> (x*y=w678:dbl)
        n437 = Number To Fractional String(number=w678) -> (F-format string=w699:string)  [unwired: 3 in]
        n438 = Number To Fractional String(number=w702) -> (F-format string=w700:string)  [unwired: 3 in]
        n439 = Concatenate Strings "Concatenate Strings"(w707, w700, "Minutos" ("string"), "\n", "Latitud es: " ("string"), w699, "\n", "Ok" ("string")) -> (w677:string)
      }
      frame 9 {
        # "Longitud total"
        # "Minutos"
        n440 = local read "Ingrese la trama completa"() -> (w750:string)
        n441 = Match Pattern(string=w750, regular expression="GGA") -> (after substring=w732:string)  [unwired: 1 in, 3 out]
        n442 = String Subset(string=w732, offset (0)=27, length (rest)=6 ("length (rest)")) -> (substring=w740:string)
        n443 = String Subset(string=w732, offset (0)=25, length (rest)=2 ("length (rest)")) -> (substring=w742:string)
        n444 = String Subset(string=w732, offset (0)=35, length (rest)=1 ("length (rest)")) -> (substring=w729:string)
        n445 = Fract/Exp String To Number(string=w740) -> (number=w739:dbl)  [unwired: 3 in, 1 out]
        n446 = Decimal String To Number(string=w742) -> (number=w741:i32)  [unwired: 2 in, 1 out]
        n447 = Equal?(x=w729, y="E") -> (x = y?=w727:bool)
        n448 = Concatenate Strings "Concatenate Strings"("+Longitud:" ("string"), "\n", w742, "grados " ("string"), "\n") -> (w736:string)
        n449 = To Double Precision Float(number=w741) -> (double precision float=w737:dbl)
        n450 = Divide(x=w739, y=60.0) -> (x/y=w723:dbl)
        n451 = Add(x=w737, y=w723) -> (x+y=w721:dbl)
        n452 = Select(t=1.0, s=w727, f=-1.0) -> (s? t:f=w724:dbl)
        n453 = Multiply(x=w721, y=w724) -> (x*y=w722:dbl)
        n454 = Number To Fractional String(number=w722) -> (F-format string=w716:string)  [unwired: 3 in]
        n455 = Number To Fractional String(number=w723) -> (F-format string=w720:string)  [unwired: 3 in]
        n456 = Concatenate Strings "Concatenate Strings"(w736, w720, "Minutos" ("string"), "\n", "Longitud es: " ("string"), w716, "\n", "Ok" ("string")) -> (w735:string)
      }
      frame 10 {
        n457 = local read "Ingrese la trama completa"() -> (w804:string)
        n458 = Match Pattern(string=w804, regular expression="GGA") -> (after substring=w800:string)  [unwired: 1 in, 3 out]
        n459 = String Subset(string=w800, offset (0)=37, length (rest)=1 ("length (rest)")) -> (substring=w752:string)
        n460 = Equal?(x=w752, y="1") -> (x = y?=w798:bool)
        n461 = Equal?(x=w752, y="0") -> (x = y?=w788:bool)
        n462 = Equal?(x=w752, y="2") -> (x = y?=w786:bool)
        n463 = Equal?(x=w752, y="3") -> (x = y?=w778:bool)
        n464 = Equal?(x=w752, y="4") -> (x = y?=w776:bool)
        n465 = Equal?(x=w752, y="5") -> (x = y?=w768:bool)
        n466 = Equal?(x=w752, y="6") -> (x = y?=w766:bool)
        n467 = Equal?(x=w752, y="7") -> (x = y?=w759:bool)
        n468 = Equal?(x=w752, y="8") -> (x = y?=w755:bool)
        n469 = Select(t=2, s=w798, f=0) -> (s? t:f=w795:i32)
        n470 = Select(t=1, s=w788, f=0) -> (s? t:f=w787:i32)
        n471 = Select(t=3, s=w786, f=0) -> (s? t:f=w782:i32)
        n472 = Select(t=4, s=w778, f=0) -> (s? t:f=w777:i32)
        n473 = Select(t=5, s=w776, f=0) -> (s? t:f=w772:i32)
        n474 = Select(t=6, s=w768, f=0) -> (s? t:f=w767:i32)
        n475 = Select(t=7, s=w766, f=0) -> (s? t:f=w762:i32)
        n476 = Select(t=8, s=w759, f=0) -> (s? t:f=w757:i32)
        n477 = Select(t=9, s=w755, f=0) -> (s? t:f=w751:i32)
        n478 = formula code="B1=(A1+A2+A3+A4\n+A5+A6+A7+A8+A9);"("A1"=w795, "A2"=w787, "A3"=w782, "A4"=w777, "A5"=w772, "A6"=w767, "A7"=w762, "A8"=w757, "A9"=w751) -> ("B1"=w794:dbl)
        n479 = To Byte Integer(number=w794) -> (8bit integer=w793:i8)
        n480 = case shown="9" w793 {
          tunnel: [w805 w811 w818 w823 w829 w835 w841 w848 w853] -> w792
          frame 2 {
            n481 = Concatenate Strings("+Capacidad de reparación: " ("string"), "\n", "1: Posición de GPS (SPS)", "\n", "Ok" ("string")) -> (w805:string)
          }
          frame 3 {
            n482 = Concatenate Strings("+Capacidad de reparación: " ("string"), "\n", " 2 : Fijo DGPS" ("string"), "\n", "Ok" ("string")) -> (w811:string)
          }
          frame 4 {
            n483 = Concatenate Strings("+Capacidad de reparación: " ("string"), "\n", "3:PPS fijo", "\n", "Ok" ("string")) -> (w818:string)
          }
          frame 5 {
            n484 = Concatenate Strings("+Capacidad de reparación: " ("string"), "\n", "4: Cinemática en tiempo real", "\n", "Ok" ("string")) -> (w823:string)
          }
          frame 6 {
            n485 = Concatenate Strings("+Capacidad de reparación: " ("string"), "\n", "5: RTK flotante", "\n", "Ok" ("string")) -> (w829:string)
          }
          frame 7 {
            n486 = Concatenate Strings("+Capacidad de reparación: " ("string"), "\n", "6: Estimado(navegación a estima)", "\n", "Ok" ("string")) -> (w835:string)
          }
          frame 8 {
            n487 = Concatenate Strings("+Capacidad de reparación: " ("string"), "\n", "7: Modo de entrada manual ", "\n", "Ok" ("string")) -> (w841:string)
          }
          frame 9 {
            n488 = Concatenate Strings("+Capacidad de reparación: " ("string"), "\n", "8: Modo de  simulación", "\n", "Ok" ("string")) -> (w848:string)
          }
          frame 1, Default {
            n489 = Concatenate Strings("+Capacidad de reparación: " ("string"), "\n", "0: No válido" ("string"), "\n", "Ok" ("string")) -> (w853:string)
          }
        }
      }
      frame 11 {
        n490 = local read "Ingrese la trama completa"() -> (w907:string)
        n491 = Match Pattern(string=w907, regular expression="GGA") -> (after substring=w861:string)  [unwired: 1 in, 3 out]
        n492 = String Subset(string=w861, offset (0)=61, length (rest)=1 ("length (rest)")) -> (substring=w866:string)
        n493 = String Subset(string=w861, offset (0)=39, length (rest)=1 ("length (rest)")) -> (substring=w901:string)
        n494 = String Subset(string=w861, offset (0)=46, length (rest)=6 ("length (rest)")) -> (substring=w886:string)
        n495 = String Subset(string=w861, offset (0)=41, length (rest)=4 ("length (rest)")) -> (substring=w892:string)
        n496 = String Subset(string=w861, offset (0)=60, length (rest)=1 ("length (rest)")) -> (substring=w870:string)
        n497 = String Subset(string=w861, offset (0)=55, length (rest)=3 ("length (rest)")) -> (substring=w878:string)
        n498 = Concatenate Strings "Concatenate Strings"("+Número de satelites en seguimiento:  " ("string"), "\n", w901, "\n") -> (w896:string)
        n499 = Concatenate Strings("+Dilución horizontal de posición:" ("string"), "\n", w892, "\n") -> (w895:string)
        n500 = Concatenate Strings("+(campo vacío) tiempo en segundos desde la última actualización de DGPS:" ("string"), "\n", w870, "\n") -> (w868:string)
        n501 = Concatenate Strings("+Altitud, Metros, sobre el nivel medio del mar:" ("string"), "\n", w886, "M" ("string"), "\n") -> (w885:string)
        n502 = Concatenate Strings("+Altura del geoide (nivel medio del mar):" ("string"), "\n", w878, "M" ("string"), "\n") -> (w875:string)
        n503 = Concatenate Strings("+(campo vacío) Número de identificación de la estación DGPS:" ("string"), "\n", w866, "\n", "Ok" ("string")) -> (w860:string)
        n504 = Concatenate Strings(w896, w895, w885, w875, w868, w860) -> (w894:string)
      }
      frame 12 {
        n505 = local read "Ingrese la trama completa"() -> (w918:string)
        n506 = Match Pattern(string=w918, regular expression="GGA") -> (after substring=w916:string)  [unwired: 1 in, 3 out]
        n507 = String Subset(string=w916, offset (0)=62, length (rest)=4 ("length (rest)")) -> (substring=w911:string)
        n508 = Concatenate Strings("+Los datos de la suma de comprobación:" ("string"), "\n", w911, "\n", "Ok" ("string")) -> (w909:string)
      }
      frame 13 {
        n509 = local read "Ingrese la trama completa"() -> (w937:string)
        n510 = Match Pattern(string=w937, regular expression="RMC") -> (after substring=w922:string)  [unwired: 1 in, 3 out]
        n511 = String Subset(string=w922, offset (0)=1, length (rest)=2 ("length (rest)")) -> (substring=w927:string)
        n512 = String Subset(string=w922, offset (0)=3, length (rest)=2 ("length (rest)")) -> (substring=w924:string)
        n513 = String Subset(string=w922, offset (0)=5, length (rest)=6 ("length (rest)")) -> (substring=w923:string)
        n514 = Concatenate Strings "Concatenate Strings"("+Hora: " ("string"), "\n", w927, ":" ("string"), w924, ":" ("string"), w923, "\n", "Ok" ("string")) -> (w919:string)
      }
      frame 14 {
        n515 = local read "Ingrese la trama completa"() -> (w953:string)
        n516 = Match Pattern(string=w953, regular expression="RMC") -> (after substring=w951:string)  [unwired: 1 in, 3 out]
        n517 = String Subset(string=w951, offset (0)=12, length (rest)=1 ("length (rest)")) -> (substring=w948:string)
        n518 = Equal?(x=w948, y="A") -> (x = y?=w946:bool)
        n519 = Select(t="A:Esta activo", s=w946, f="V: Sin señal") -> (s? t:f=w943:string)
        n520 = Concatenate Strings("+Estado:" ("string"), "\n", w943, "\n", "Ok" ("string")) -> (w940:string)
      }
      frame 15 {
        # "Latitud total"
        # "Minutos"
        n521 = local read "Ingrese la trama completa"() -> (w990:string)
        n522 = Match Pattern(string=w990, regular expression="RMC") -> (after substring=w973:string)  [unwired: 1 in, 3 out]
        n523 = String Subset(string=w973, offset (0)=15, length (rest)=2 ("length (rest)")) -> (substring=w982:string)
        n524 = String Subset(string=w973, offset (0)=17, length (rest)=6 ("length (rest)")) -> (substring=w977:string)
        n525 = String Subset(string=w973, offset (0)=24, length (rest)=1 ("length (rest)")) -> (substring=w970:string)
        n526 = Decimal String To Number(string=w982) -> (number=w981:i32)  [unwired: 2 in, 1 out]
        n527 = Fract/Exp String To Number(string=w977) -> (number=w976:dbl)  [unwired: 3 in, 1 out]
        n528 = Equal?(x=w970, y="N") -> (x = y?=w968:bool)
        n529 = Concatenate Strings "Concatenate Strings"("+Latitud:" ("string"), "\n", w982, "grados " ("string"), "\n") -> (w964:string)
        n530 = To Double Precision Float(number=w981) -> (double precision float=w980:dbl)
        n531 = Divide(x=w976, y=60.0) -> (x/y=w963:dbl)
        n532 = Add(x=w980, y=w963) -> (x+y=w974:dbl)
        n533 = Select(t=1.0, s=w968, f=-1.0) -> (s? t:f=w965:dbl)
        n534 = Multiply(x=w974, y=w965) -> (x*y=w956:dbl)
        n535 = Number To Fractional String(number=w956) -> (F-format string=w958:string)  [unwired: 3 in]
        n536 = Number To Fractional String(number=w963) -> (F-format string=w962:string)  [unwired: 3 in]
        n537 = Concatenate Strings(w964, w962, "Minutos " ("string"), "\n", "La latitud es: " ("string"), w958, "\n", "Ok " ("string")) -> (w955:string)
      }
      frame 16 {
        # "Longitud total"
        # "Minutos"
        n538 = local read "Ingrese la trama completa"() -> (w1027:string)
        n539 = Match Pattern(string=w1027, regular expression="RMC") -> (after substring=w1014:string)  [unwired: 1 in, 3 out]
        n540 = String Subset(string=w1014, offset (0)=29, length (rest)=6 ("length (rest)")) -> (substring=w1019:string)
        n541 = String Subset(string=w1014, offset (0)=27, length (rest)=2 ("length (rest)")) -> (substring=w1023:string)
        n542 = String Subset(string=w1014, offset (0)=37, length (rest)=1 ("length (rest)")) -> (substring=w1011:string)
        n543 = Fract/Exp String To Number(string=w1019) -> (number=w1018:dbl)  [unwired: 3 in, 1 out]
        n544 = Decimal String To Number(string=w1023) -> (number=w1022:i32)  [unwired: 2 in, 1 out]
        n545 = Equal?(x=w1011, y="E") -> (x = y?=w1009:bool)
        n546 = Concatenate Strings("+Longitud: " ("string"), "\n", w1023, "grados " ("string"), "\n") -> (w1004:string)
        n547 = Select(t=1.0, s=w1009, f=-1.0) -> (s? t:f=w1006:dbl)
        n548 = Divide(x=w1018, y=60.0) -> (x/y=w998:dbl)
        n549 = Number To Fractional String(number=w998) -> (F-format string=w1003:string)  [unwired: 3 in]
        n550 = To Double Precision Float(number=w1022) -> (double precision float=w1016:dbl)
        n551 = Add(x=w1016, y=w998) -> (x+y=w1015:dbl)
        n552 = Multiply(x=w1015, y=w1006) -> (x*y=w1005:dbl)
        n553 = Number To Fractional String(number=w1005) -> (F-format string=w999:string)  [unwired: 3 in]
        n554 = Concatenate Strings(w1004, w1003, "Minutos" ("string"), "\n", "Longitud es: " ("string"), w999, "\n", "Ok" ("string")) -> (w997:string)
      }
      frame 17 {
        n555 = local read "Ingrese la trama completa"() -> (w1038:string)
        n556 = Match Pattern(string=w1038, regular expression="RMC") -> (after substring=w1036:string)  [unwired: 1 in, 3 out]
        n557 = String Subset(string=w1036, offset (0)=39, length (rest)=4 ("length (rest)")) -> (substring=w1031:string)
        n558 = Concatenate Strings("+Velocidad:" ("string"), "\n", w1031, "\n", "Ok" ("string")) -> (w1028:string)
      }
      frame 18 {
        n559 = local read "Ingrese la trama completa"() -> (w1049:string)
        n560 = Match Pattern(string=w1049, regular expression="RMC") -> (after substring=w1047:string)  [unwired: 1 in, 3 out]
        n561 = String Subset(string=w1047, offset (0)=44, length (rest)=6 ("length (rest)")) -> (substring=w1042:string)
        n562 = Concatenate Strings("+Angulo:" ("string"), "\n", w1042, "\n", "Ok" ("string")) -> (w1039:string)
      }
      frame 19 {
        n563 = local read "Ingrese la trama completa"() -> (w1068:string)
        n564 = Match Pattern(string=w1068, regular expression="RMC") -> (after substring=w1062:string)  [unwired: 1 in, 3 out]
        n565 = String Subset(string=w1062, offset (0)=51, length (rest)=2 ("length (rest)")) -> (substring=w1057:string)
        n566 = String Subset(string=w1062, offset (0)=53, length (rest)=2 ("length (rest)")) -> (substring=w1055:string)
        n567 = String Subset(string=w1062, offset (0)=55, length (rest)=2 ("length (rest)")) -> (substring=w1053:string)
        n568 = Concatenate Strings "Concatenate Strings"("+Fecha:" ("string"), "\n", w1057, "/" ("string"), w1055, "/" ("string"), w1053, "\n", "Ok" ("string")) -> (w1052:string)
      }
      frame 20 {
        n569 = local read "Ingrese la trama completa"() -> (w1079:string)
        n570 = Match Pattern(string=w1079, regular expression="RMC") -> (after substring=w1077:string)  [unwired: 1 in, 3 out]
        n571 = String Subset(string=w1077, offset (0)=57, length (rest)=6 ("length (rest)")) -> (substring=w1072:string)
        n572 = Concatenate Strings "Concatenate Strings"("+Variación magnéctica: " ("string"), "\n", w1072, "\n", "Ok" ("string")) -> (w1071:string)
      }
      frame 21 {
        n573 = local read "Ingrese la trama completa"() -> (w1090:string)
        n574 = Match Pattern(string=w1090, regular expression="RMC") -> (after substring=w1088:string)  [unwired: 1 in, 3 out]
        n575 = String Subset(string=w1088, offset (0)=63, length (rest)=3 ("length (rest)")) -> (substring=w1083:string)
        n576 = Concatenate Strings "Concatenate Strings"("+Suma de comprobación: " ("string"), "\n", w1083, "\n", "Ok" ("string")) -> (w1080:string)
      }
      frame 22 {
        n577 = local read "Ingrese la trama completa"() -> (w1106:string)
        n578 = Match Pattern(string=w1106, regular expression="GSA") -> (after substring=w1104:string)  [unwired: 1 in, 3 out]
        n579 = String Subset(string=w1104, offset (0)=1, length (rest)=1 ("length (rest)")) -> (substring=w1097:string)
        n580 = Equal?(x=w1097, y="A") -> (x = y?=w1100:bool)
        n581 = Select(t="A:Esta activo", s=w1100, f="V: Sin señal") -> (s? t:f=w1096:string)
        n582 = Concatenate Strings "Concatenate Strings"("+Estado:" ("string"), "\n", w1096, "\n", "Ok" ("string")) -> (w1093:string)
      }
      frame 23 {
        n583 = local read "Ingrese la trama completa"() -> (w1130:string)
        n584 = Match Pattern(string=w1130, regular expression="GSA") -> (after substring=w1128:string)  [unwired: 1 in, 3 out]
        n585 = String Subset(string=w1128, offset (0)=3, length (rest)=1 ("length (rest)")) -> (substring=w1123:string)
        n586 = Equal?(x=w1123, y="1") -> (x = y?=w1121:bool)
        n587 = Equal?(x=w1123, y="2") -> (x = y?=w1118:bool)
        n588 = Equal?(x=w1123, y="3") -> (x = y?=w1115:bool)
        n589 = Select(t=1, s=w1121, f=0) -> (s? t:f=w1112:i32)
        n590 = Select(t=2, s=w1118, f=0) -> (s? t:f=w1111:i32)
        n591 = Select(t=3, s=w1115, f=0) -> (s? t:f=w1110:i32)
        n592 = formula code="B2=(A9+A10+A11);"("A9"=w1112, "A10"=w1111, "A11"=w1110) -> ("B2"=w1108:dbl)
        n593 = To Byte Integer(number=w1108) -> (8bit integer=w1109:i8)
        n594 = case shown="1" w1109 {
          tunnel: ["" w1132 w1138 w1144] -> w1107
          frame 0, Default {
          }
          frame 1 {
            n595 = Concatenate Strings("+Selección automática de corección: " ("string"), "\n", "1:Sin correccción" ("string"), "\n", "Ok" ("string")) -> (w1132:string)
          }
          frame 2 {
            n596 = Concatenate Strings("+Selección automática de corección: " ("string"), "\n", "2:Arreglo 2D" ("string"), "\n", "Ok" ("string")) -> (w1138:string)
          }
          frame 3 {
            n597 = Concatenate Strings("+Selección automática de corección: " ("string"), "\n", "3: Corrección 3D" ("string"), "\n", "Ok" ("string")) -> (w1144:string)
          }
        }
      }
      frame 24 {
        n598 = local read "Ingrese la trama completa"() -> (w1176:string)
        n599 = Match Pattern(string=w1176, regular expression="GSA") -> (after substring=w1156:string)  [unwired: 1 in, 3 out]
        n600 = String Subset(string=w1156, offset (0)=14, length (rest)=2 ("length (rest)")) -> (substring=w1158:string)
        n601 = String Subset(string=w1156, offset (0)=11, length (rest)=2 ("length (rest)")) -> (substring=w1160:string)
        n602 = String Subset(string=w1156, offset (0)=8, length (rest)=2 ("length (rest)")) -> (substring=w1162:string)
        n603 = String Subset(string=w1156, offset (0)=5, length (rest)=2 ("length (rest)")) -> (substring=w1164:string)
        n604 = String Subset(string=w1156, offset (0)=17, length (rest)=2 ("length (rest)")) -> (substring=w1153:string)
        n605 = Concatenate Strings "Concatenate Strings"("+PRN de satelites utilizados para fijar: " ("string"), "\n", w1164, "," ("string"), w1162, "," ("string"), w1160, "," ("string"), w1158, "," ("string"), w1153, "\n", "Ok" ("string")) -> (w1157:string)
      }
      frame 25 {
        n606 = local read "Ingrese la trama completa"() -> (w1199:string)
        n607 = Match Pattern(string=w1199, regular expression="GSA") -> (after substring=w1193:string)  [unwired: 1 in, 3 out]
        n608 = String Subset(string=w1193, offset (0)=37, length (rest)=4 ("length (rest)")) -> (substring=w1180:string)
        n609 = String Subset(string=w1193, offset (0)=32, length (rest)=4 ("length (rest)")) -> (substring=w1184:string)
        n610 = String Subset(string=w1193, offset (0)=27, length (rest)=4 ("length (rest)")) -> (substring=w1188:string)
        n611 = Concatenate Strings("+PDOP (dilución de precisión):" ("string"), "\n", w1188, "\n", "+Dilución horizontal de precisión (HDOP):" ("string"), "\n", w1184, "\n", "+Dilución vertical de precisión (VDOP):" ("string"), "\n", w1180, "\n", "Ok" ("string")) -> (w1177:string)
      }
      frame 26 {
        n612 = local read "Ingrese la trama completa"() -> (w1210:string)
        n613 = Match Pattern(string=w1210, regular expression="GSA") -> (after substring=w1206:string)  [unwired: 1 in, 3 out]
        n614 = String Subset(string=w1206, offset (0)=42, length (rest)=4 ("length (rest)")) -> (substring=w1203:string)
        n615 = Concatenate Strings "Concatenate Strings"("+Suma de comprobación:" ("string"), "\n", w1203, "\n", "Ok" ("string")) -> (w1202:string)
      }
      frame 27 {
        n616 = Get Date/Time In Seconds() -> (seconds since 1Jan1904=w1217:timestamp)
        n617 = Get Date/Time String(seconds (now)=w1217) -> (time string=w1214:string)  [unwired: 2 in, 1 out]
        n618 = Concatenate Strings "Concatenate Strings"("+Reloj:" ("string"), "\n", w1214, "\n", "Ok" ("string")) -> (w1211:string)
      }
      frame 28 {
        n619 = Get Date/Time In Seconds() -> (seconds since 1Jan1904=w1224:timestamp)
        n620 = Get Date/Time String(seconds (now)=w1224) -> (date string=w1222:string)  [unwired: 2 in, 1 out]
        n621 = Concatenate Strings "Concatenate Strings"("+Fecha:" ("string"), "\n", w1222, "\n", "Ok" ("string")) -> (w1218:string)
      }
      frame 29 {
        n622 = Concatenate Strings "Concatenate Strings"("+Bateria:" ("string"), "\n", "Op1:(0-3,3V); Op2:(0-100V)" ("string"), "\n", "Ok" ("string")) -> (w1225:string)
      }
      frame 30 {
        n623 = Concatenate Strings "Concatenate Strings"("+Bateria: 3,3V" ("string"), "\n", "Ok" ("string")) -> (w1231:string)
      }
      frame 31 {
        n624 = Concatenate Strings "Concatenate Strings"("+Bateria: 100V", "\n", "Ok" ("string")) -> (w1235:string)
      }
      frame 32 {
        n625 = local read "El contador se encuentra"() -> (w1242:dbl)
        n626 = Number To Fractional String(number=w1242, precision (6)=i16 1) -> (F-format string=w1247:string)  [unwired: 2 in]
        n627 = Concatenate Strings "Concatenate Strings"("+Contador esta:" ("string"), "\n", w1247, "Segundos" ("string"), "\n", "Ok" ("string")) -> (w1243:string)
      }
      frame 33 {
        n628 = local read "Respuesta de comandos"() -> (w1253:string)
        n629 = Decimal String To Number(string=w1253) -> (number=→"Visualizador del tiempo del contador en ms":i32)  [unwired: 2 in, 1 out]
        n630 = Concatenate Strings "Concatenate Strings"("+Respuesta de comandos:" ("string"), "\n", w1253, "ms" ("string"), "\n", "OK") -> (w1254:string)
      }
      frame 34 {
        n631 = local read "Ingrese comando"() -> (w1263:string)
        n632 = Match Pattern(string=w1263, regular expression=":") -> (after substring=w1258:string)  [unwired: 1 in, 3 out]
        n633 = Match Pattern(string=w1258, regular expression=",") -> (after substring=w1256:string)  [unwired: 1 in, 3 out]
        n634 = Concatenate Strings "Concatenate Strings"("+El parámetro a buscar y la respuesta del comando es: " ("string"), "\n", w1256, "\n", "Ok" ("string")) -> (w1264:string)
      }
      frame 35 {
        # "Selecciona operación switche"
        # "Selecciona comando"
        n635 = local read "Ingrese comando"() -> (w1266:string)
        n636 = To Upper Case(1:w1266) -> (0:w1267:string)
        n637 = Match Pattern(string=w1267, regular expression=":") -> (after substring=w1273:string)  [unwired: 1 in, 3 out]
        n638 = String Subset(string=w1273, offset (0)=0, length (rest)=2 ("length (rest)")) -> (substring=w1272:string)
        n639 = Equal?(x=w1272, y="CO") -> (x = y?=w1275:bool)
        n640 = Select(t=TRUE, s=w1275, f=FALSE) -> (s? t:f=w1270:bool)
        "SW/CO" <- w1270
        n641 = case shown="False" w1270 {
          tunnel: w1267 -> [_ w1339]
          tunnel: w1267 -> [_ w1332]
          tunnel: w1267 -> [_ w1325]
          tunnel: [w1282 ""] -> w1269
          frame False {
            n642 = local read "Led Uno"() -> (w1310:bool)
            n643 = local read "Led Dos"() -> (w1309:bool)
            n644 = local read "Led Tres"() -> (w1308:bool)
            n645 = Equal?(x=w1310, y=TRUE) -> (x = y?=w1319:bool)
            n646 = Equal?(x=w1308, y=TRUE) -> (x = y?=w1315:bool)
            n647 = Equal?(x=w1309, y=TRUE) -> (x = y?=w1316:bool)
            n648 = Select(t="Led2 ON", s=w1316, f="Led2 OFF") -> (s? t:f=w1317:string)
            n649 = Select(t="Led1 ON", s=w1319, f="Led1 OFF") -> (s? t:f=w1318:string)
            n650 = Select(t="Led3 ON", s=w1315, f="Led3 OFF") -> (s? t:f=w1314:string)
            n651 = Concatenate Strings "Concatenate Strings"("+Led Tres:" ("string"), "\n", w1314, "\n", "Ok" ("string")) -> (w1311:string)
            n652 = Concatenate Strings "Concatenate Strings"("+Led dos:" ("string"), "\n", w1317, "\n", "Ok" ("string")) -> (w1312:string)
            n653 = Concatenate Strings "Concatenate Strings"("+Led uno:" ("string"), "\n", w1318, "\n", "Ok" ("string")) -> (w1313:string)
            n654 = Concatenate Strings("+Estado de los tres leds" ("string"), "\n", w1313, "\n", w1312, "\n", w1311, "\n", "Ok" ("string")) -> (w1282:string)
          }
          frame True {
            n655 = Match Pattern(string=w1325, regular expression="LED1") -> (after substring=w1350:string)  [unwired: 1 in, 3 out]
            n656 = Match Pattern(string=w1332, regular expression="LED2") -> (after substring=w1346:string)  [unwired: 1 in, 3 out]
            n657 = Match Pattern(string=w1339, regular expression="LED3") -> (after substring=w1347:string)  [unwired: 1 in, 3 out]
            n658 = String Subset(string=w1346, offset (0)=1, length (rest)=2 ("length (rest)")) -> (substring=w1353:string)
            n659 = String Subset(string=w1347, offset (0)=1, length (rest)=2 ("length (rest)")) -> (substring=w1352:string)
            n660 = String Subset(string=w1350, offset (0)=1, length (rest)=2 ("length (rest)")) -> (substring=w1351:string)
            n661 = Equal?(x=w1351, y="ON") -> (x = y?=w1342:bool)
            n662 = Equal?(x=w1353, y="ON") -> (x = y?=w1345:bool)
            n663 = Equal?(x=w1352, y="ON") -> (x = y?=w1348:bool)
            n664 = Select(t=TRUE, s=w1345, f=FALSE) -> (s? t:f=→"LED2":bool)
            n665 = Select(t=TRUE, s=w1342, f=FALSE) -> (s? t:f=→"LED1":bool)
            n666 = Select(t=TRUE, s=w1348, f=FALSE) -> (s? t:f=→"LED3":bool)
          }
        }
        n667 = Concatenate Strings(w1269) -> (w1268:string)
      }
    }
    "Respuesta de comandos" <- w228
  }
